vi "A170316-11_Auto -ECU.vi"() -> ()   [LabVIEW 2020]
uses:
  2e0b5f5e-2208-4490-a798-25a802626be8.vi
  Global_Variable/A170316-11.vi
  Global_Variable/Global.vi
  Database/Global1.vi
  <vilib>/addons/database/Connection.llb/DB Tools Open Connec (String).vi
  <vilib>/addons/database/NI_Database_API.lvlib
  <vilib>/regexp/Match Regular Expression.xnode
panel:
  out "请拾取O型圈":bool
  out "请拾取弹簧":bool
  in  "控制器支架":T1(ring)
  in  "ECU步骤":T2(ring)
  in  "电机步骤":T3(ring)
  out "产品型号":string
  in  "更换产品":refnum<vi>
  in  "前序OK？_ECU":string
  in  "前序OK？":string
  in  "Process":string[](array[string])
  in  "Code":string[](array[string])
  in  "User":string[](array[string])
  in  "Result":string[](array[string])
  in  "Device":string[](array[string])
  out "安装支架螺栓4拧紧确认":bool
  in  "STEP2":string
  in  "STEP1":string
  out "控制器安装螺栓3拧紧确认":bool
  out "电机安装螺栓3扭矩确认":bool
  out "控制器支架螺栓5拧紧确认":bool
  out "安装扎带并取走工件":bool
  out "涂色标":bool
  out "按启动按钮拍照确认":bool
  out "电机安装螺栓2扭矩确认":bool
  out "电机安装螺栓1扭矩确认":bool
  out "安装支架涂色标":bool
  out "控制器安装螺栓2拧紧确认":bool
  out "控制器安装螺栓1拧紧确认":bool
  out "安装支架螺栓2拧紧确认":bool
  out "安装弹性垫圈弹簧并按启动拍照":bool
  out "安装支架螺栓1拧紧确认":bool
  out "控制器支架涂色标":bool
  out "控制器支架螺栓4拧紧确认":bool
  out "控制器支架螺栓3拧紧确认":bool
  out "控制器支架螺栓2拧紧确认":bool
  out "控制器支架螺栓1拧紧确认":bool
  out "安装支架螺栓3拧紧确认":bool
  in  "更换布局":string
  out "安装扎带和线卡并取走工件":bool
  out "安装支架扎带安装":bool
  out "安装支架线卡扎带安装":bool
  out "控制器支架安装线卡扎带":bool
  out "磨合次数":i32
  in  "判定结果":bool[][](array[boolean])=[[TRUE]]
  in  "STEP3":string
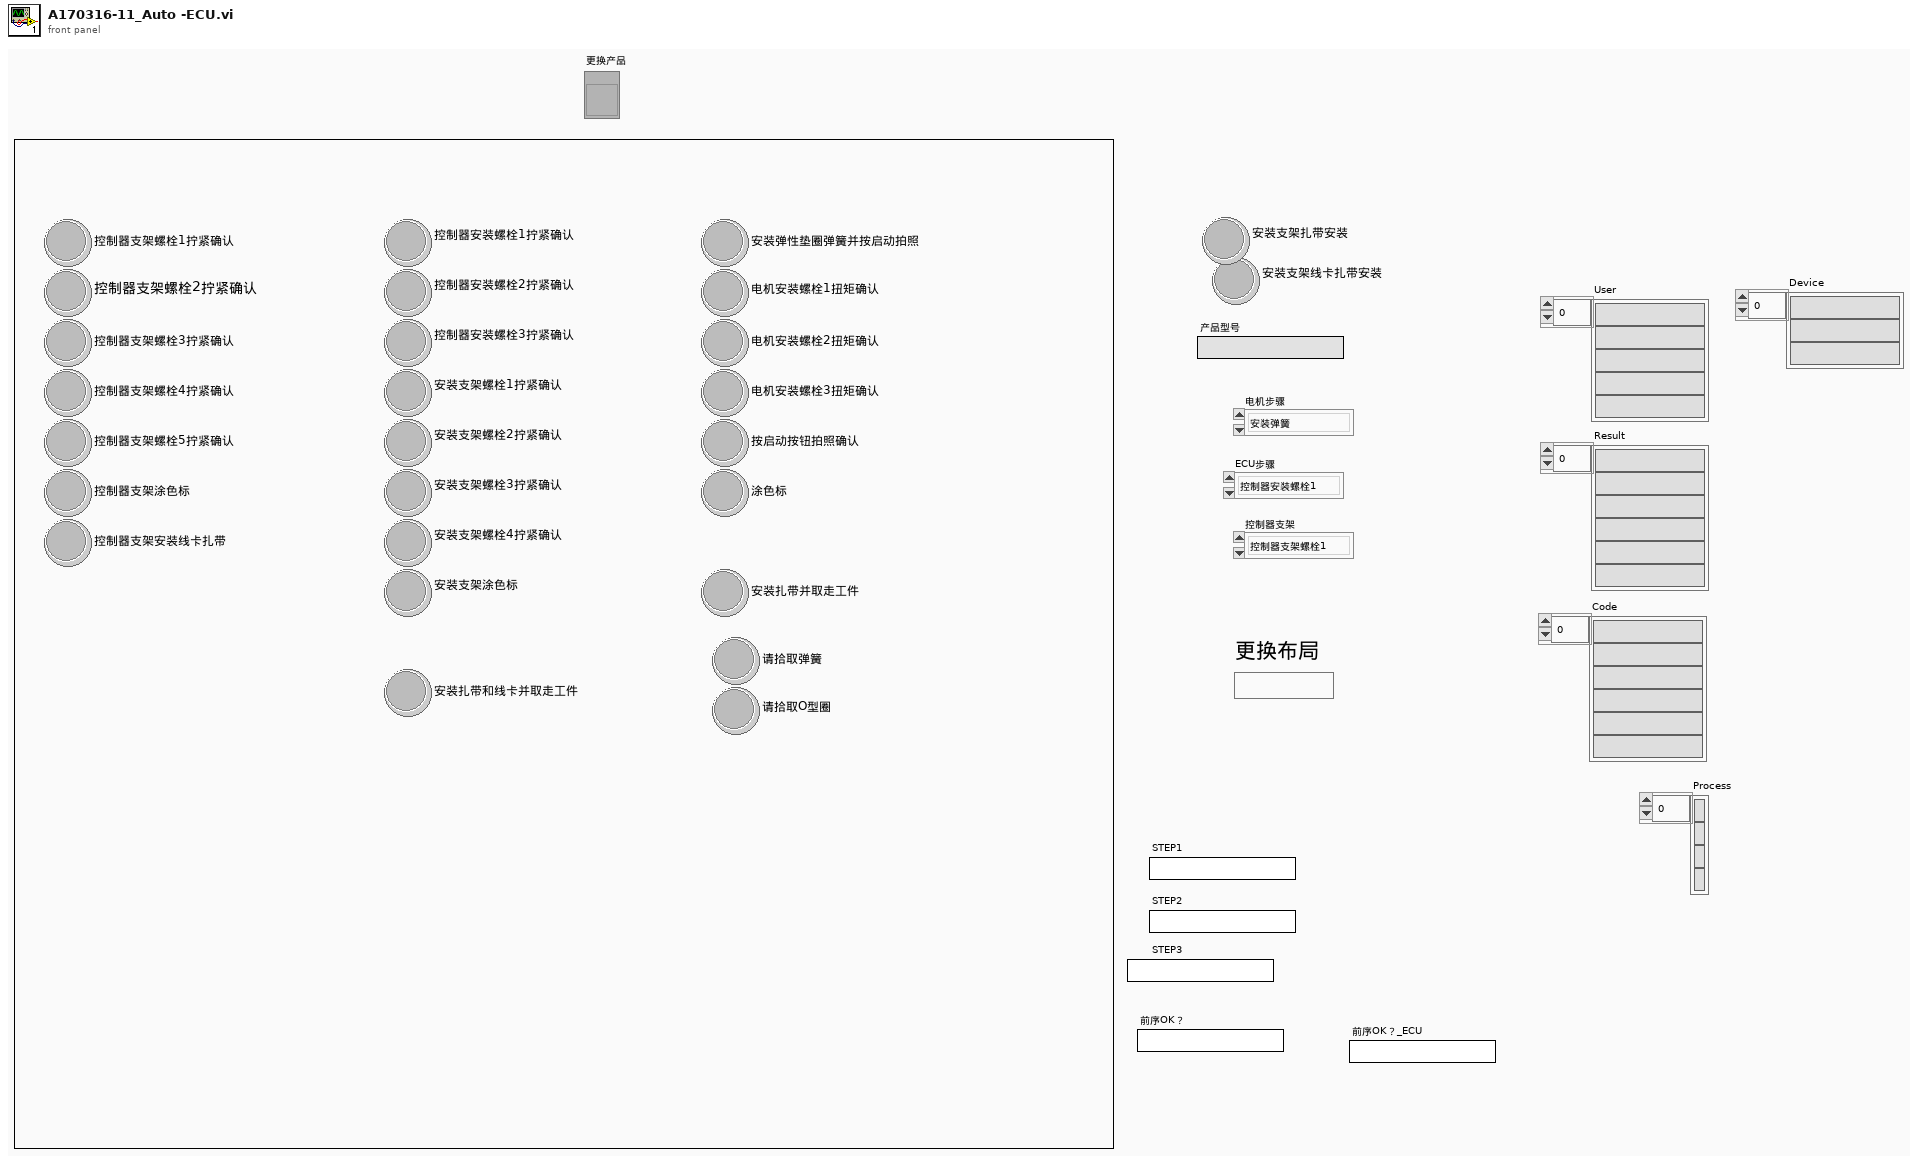
[diagram p1: front panel]
types:
  T1 = enum16{"控制器支架螺栓1", "控制器支架螺栓2", "控制器支架螺栓3", "控制器支架螺栓4", "控制器支架螺栓5", "涂色标", "安装线卡轧带", "完成"}
  T2 = enum16{"控制器安装螺栓1", "控制器安装螺栓2", "控制器安装螺栓3", "安装支架螺栓1", "安装支架螺栓2", "安装支架螺栓3", "安装支架螺栓4", "涂色标", "安装线卡取走工件", "完成"}
  T3 = enum16{"安装弹簧", "安装O型圈", "安装弹性垫圈", "电机螺栓1", "电机螺栓2", "电机螺栓3", "电机拍照", "涂色标", "安装轧带取走工件", "完成"}
  T4 = cluster{i64, i64, i64, "ECU工位生产结果":string, "result string":string}
  T5 = cluster{i64, i64, i64, "ECU工位生产结果":string, "result string":string}[]
  T6 = typedef "NI_Database_API.lvlib/Conn ObjectReference.ctl" = refnum<k1>
  T7 = cluster{"ECU工位生产结果":string, "result string":string}
  T8 = cluster{i64, i64, i64, "电机工位生产结果":string, "result string":string}
  T9 = cluster{i64, i64, i64, "电机工位生产结果":string, "result string":string}[]
  T10 = cluster{"电机工位生产结果":string, "result string":string}
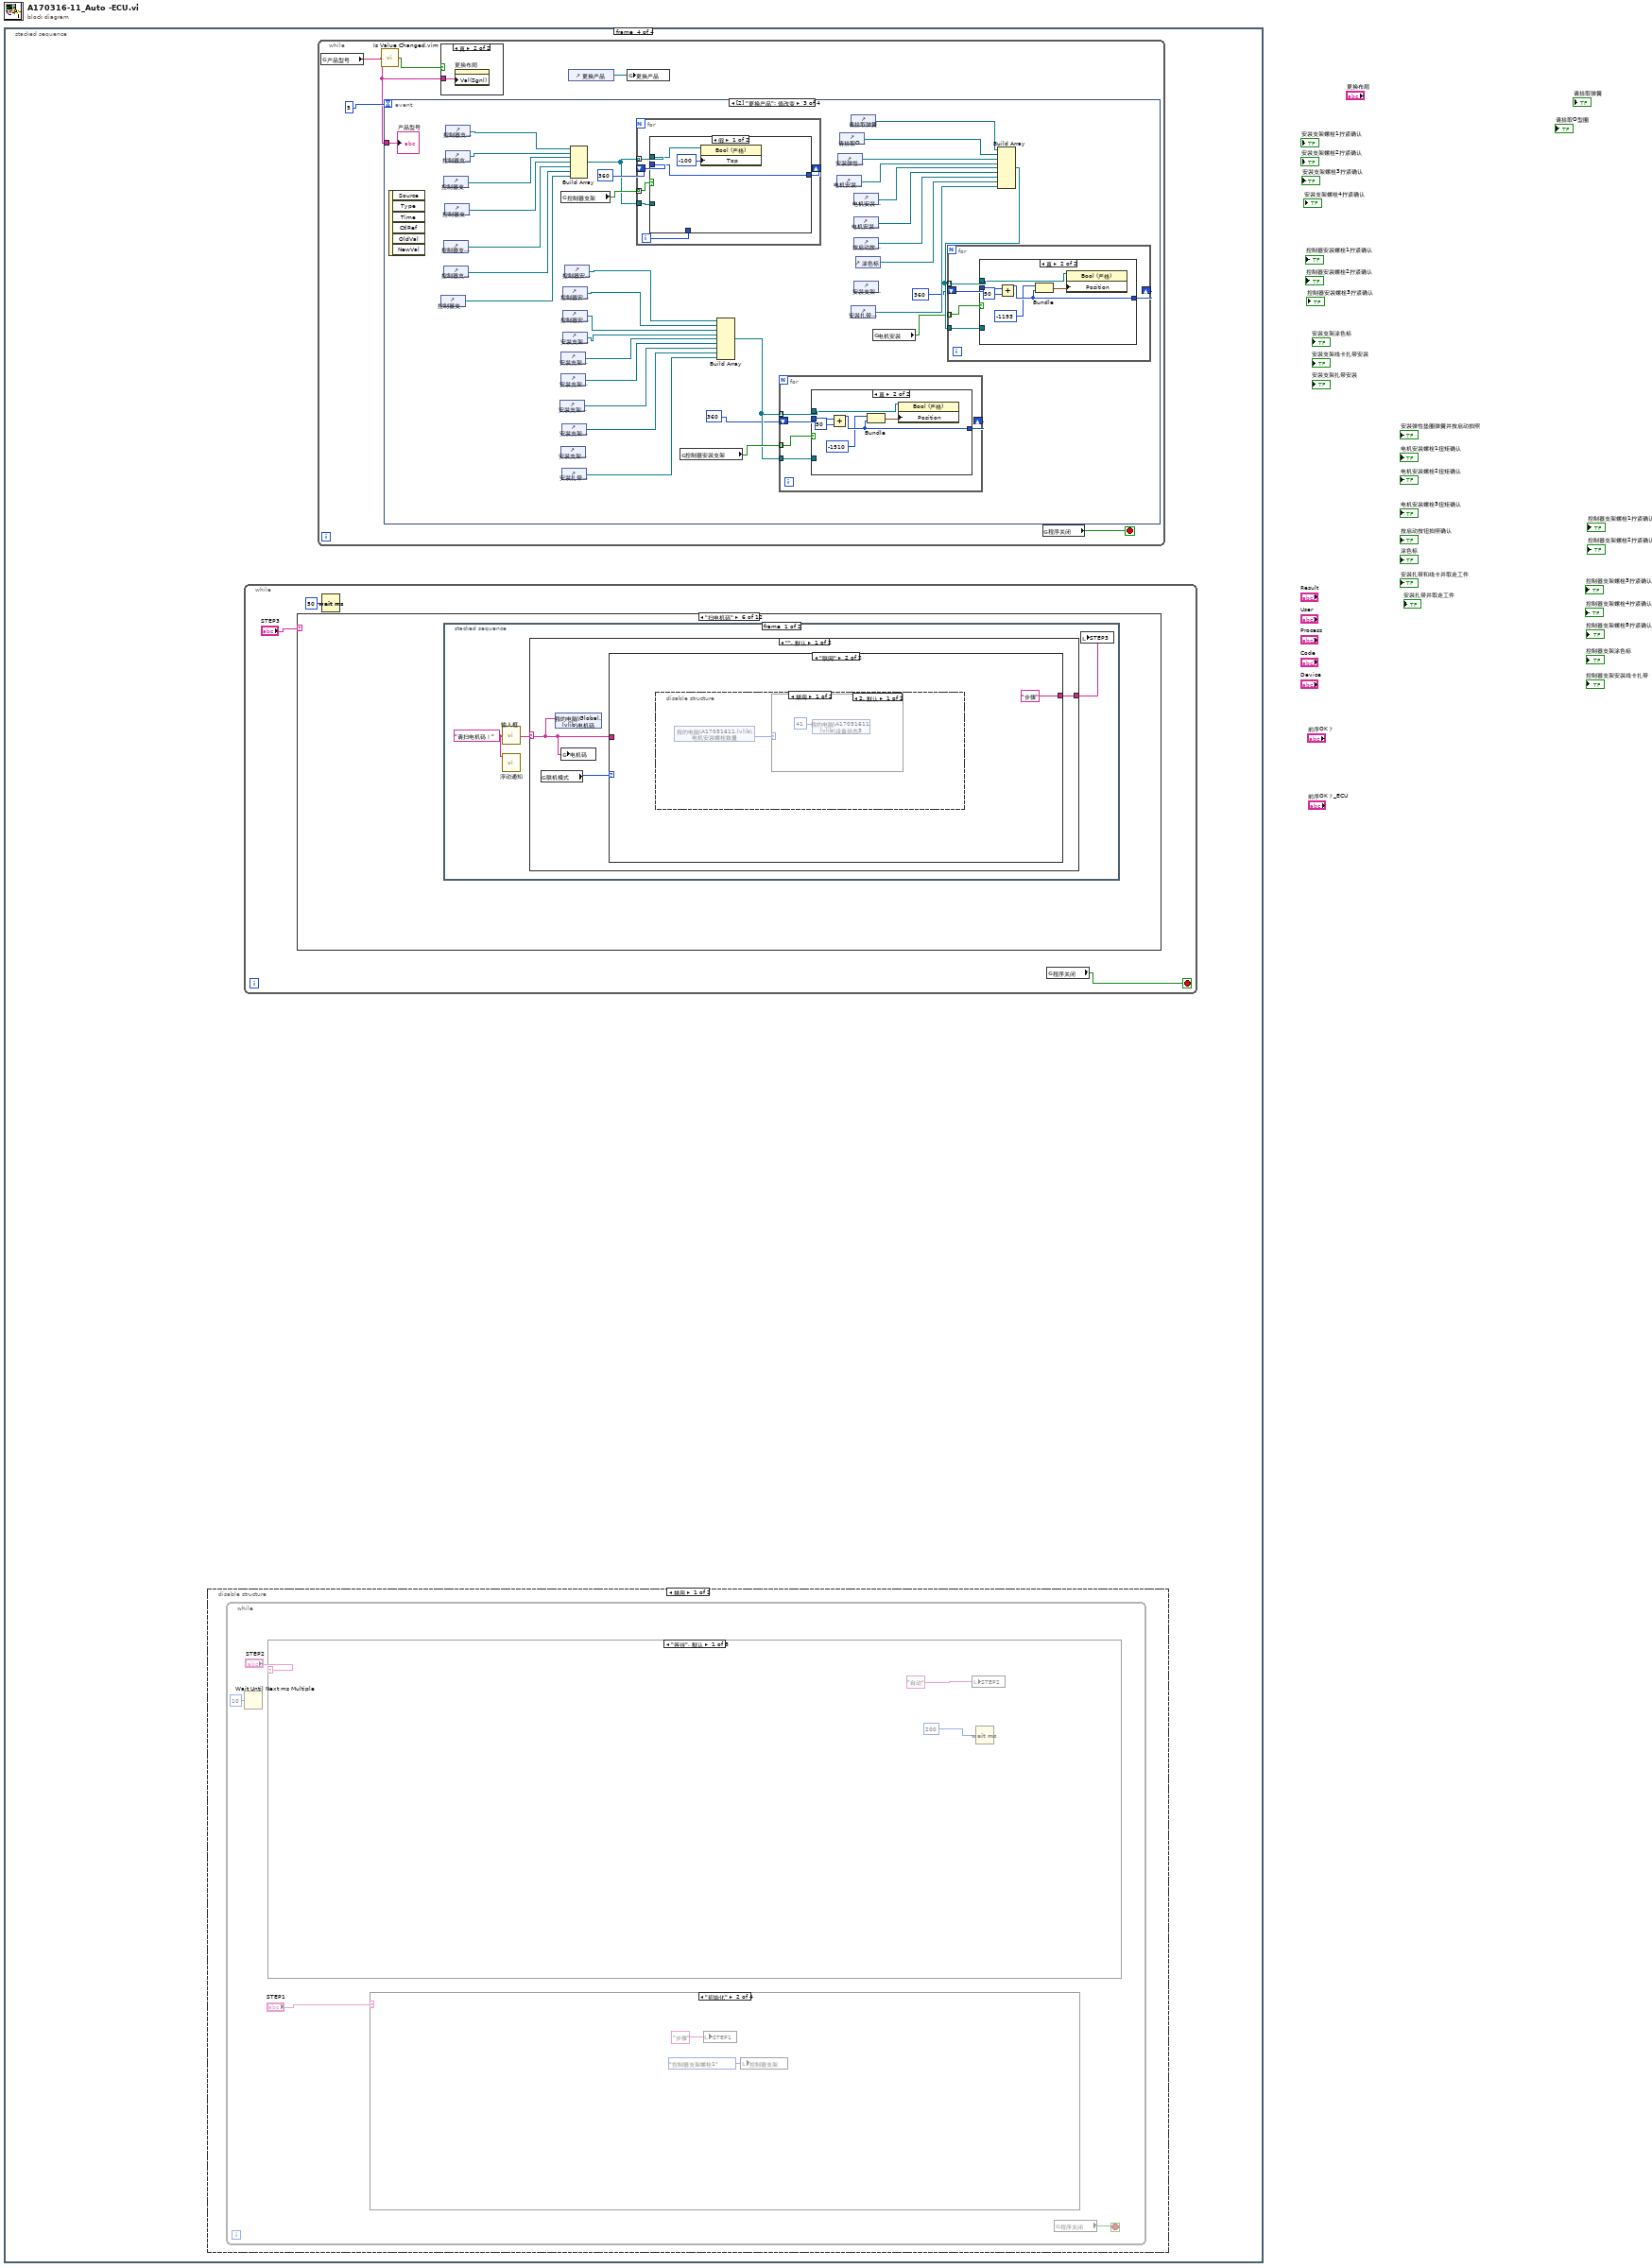
[diagram p0: block diagram]
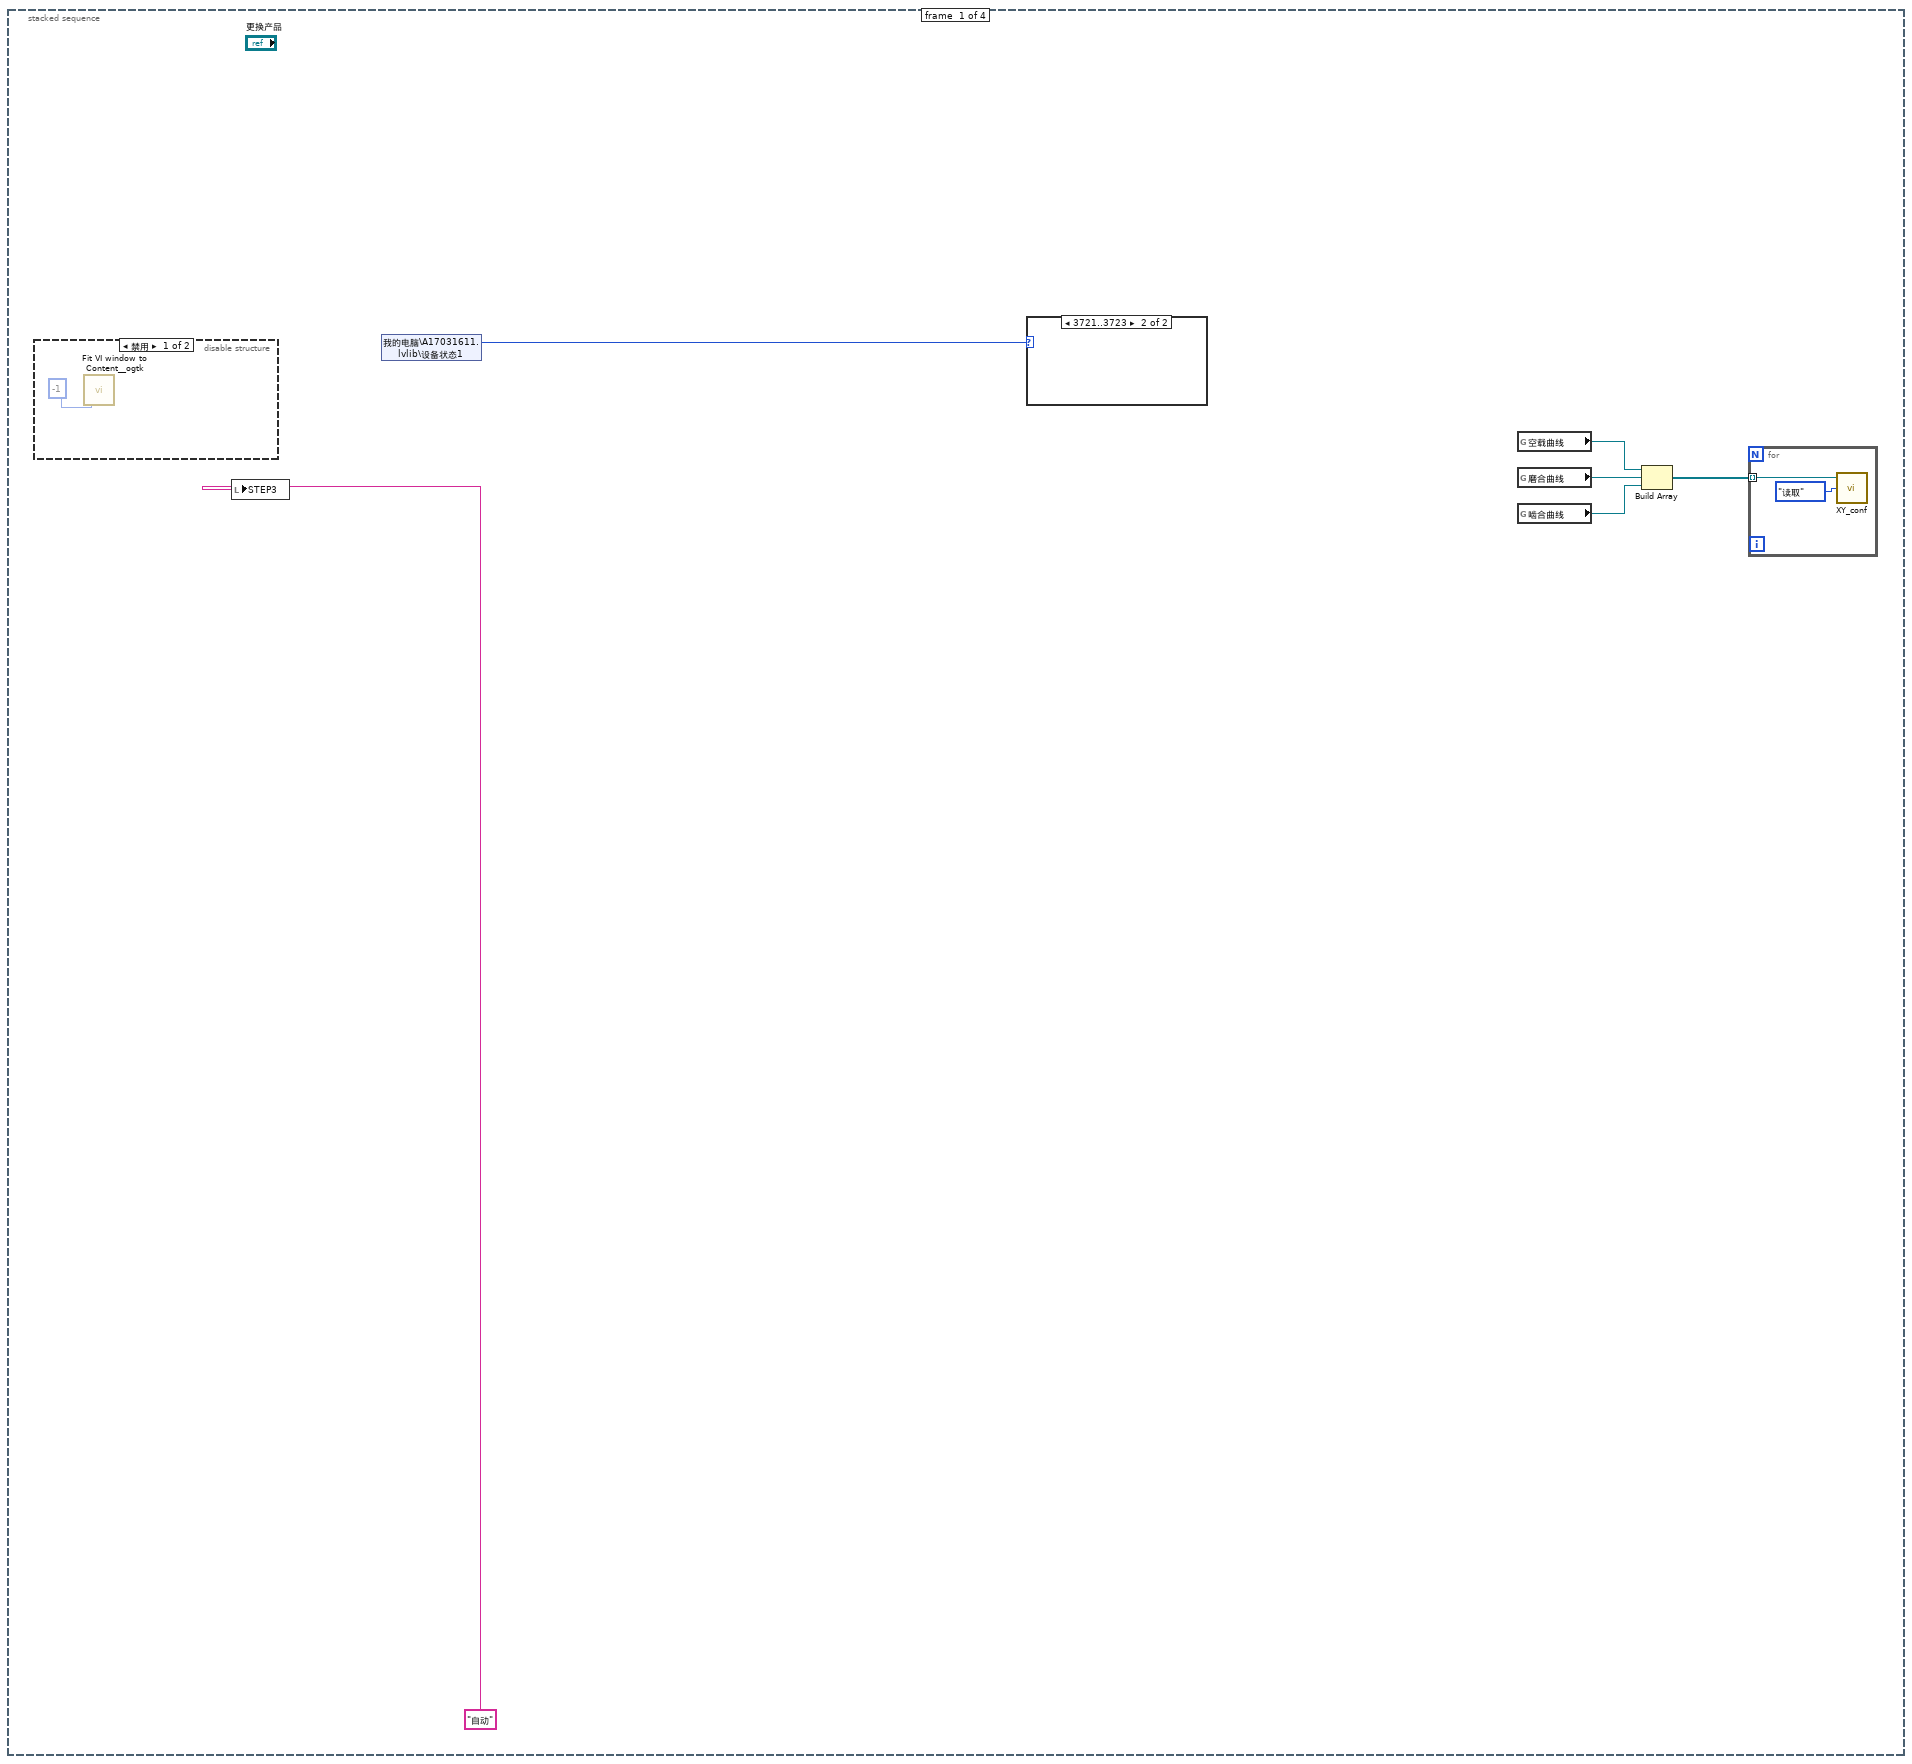
[diagram p2: hidden frame]
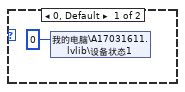
[diagram p4: hidden frame]
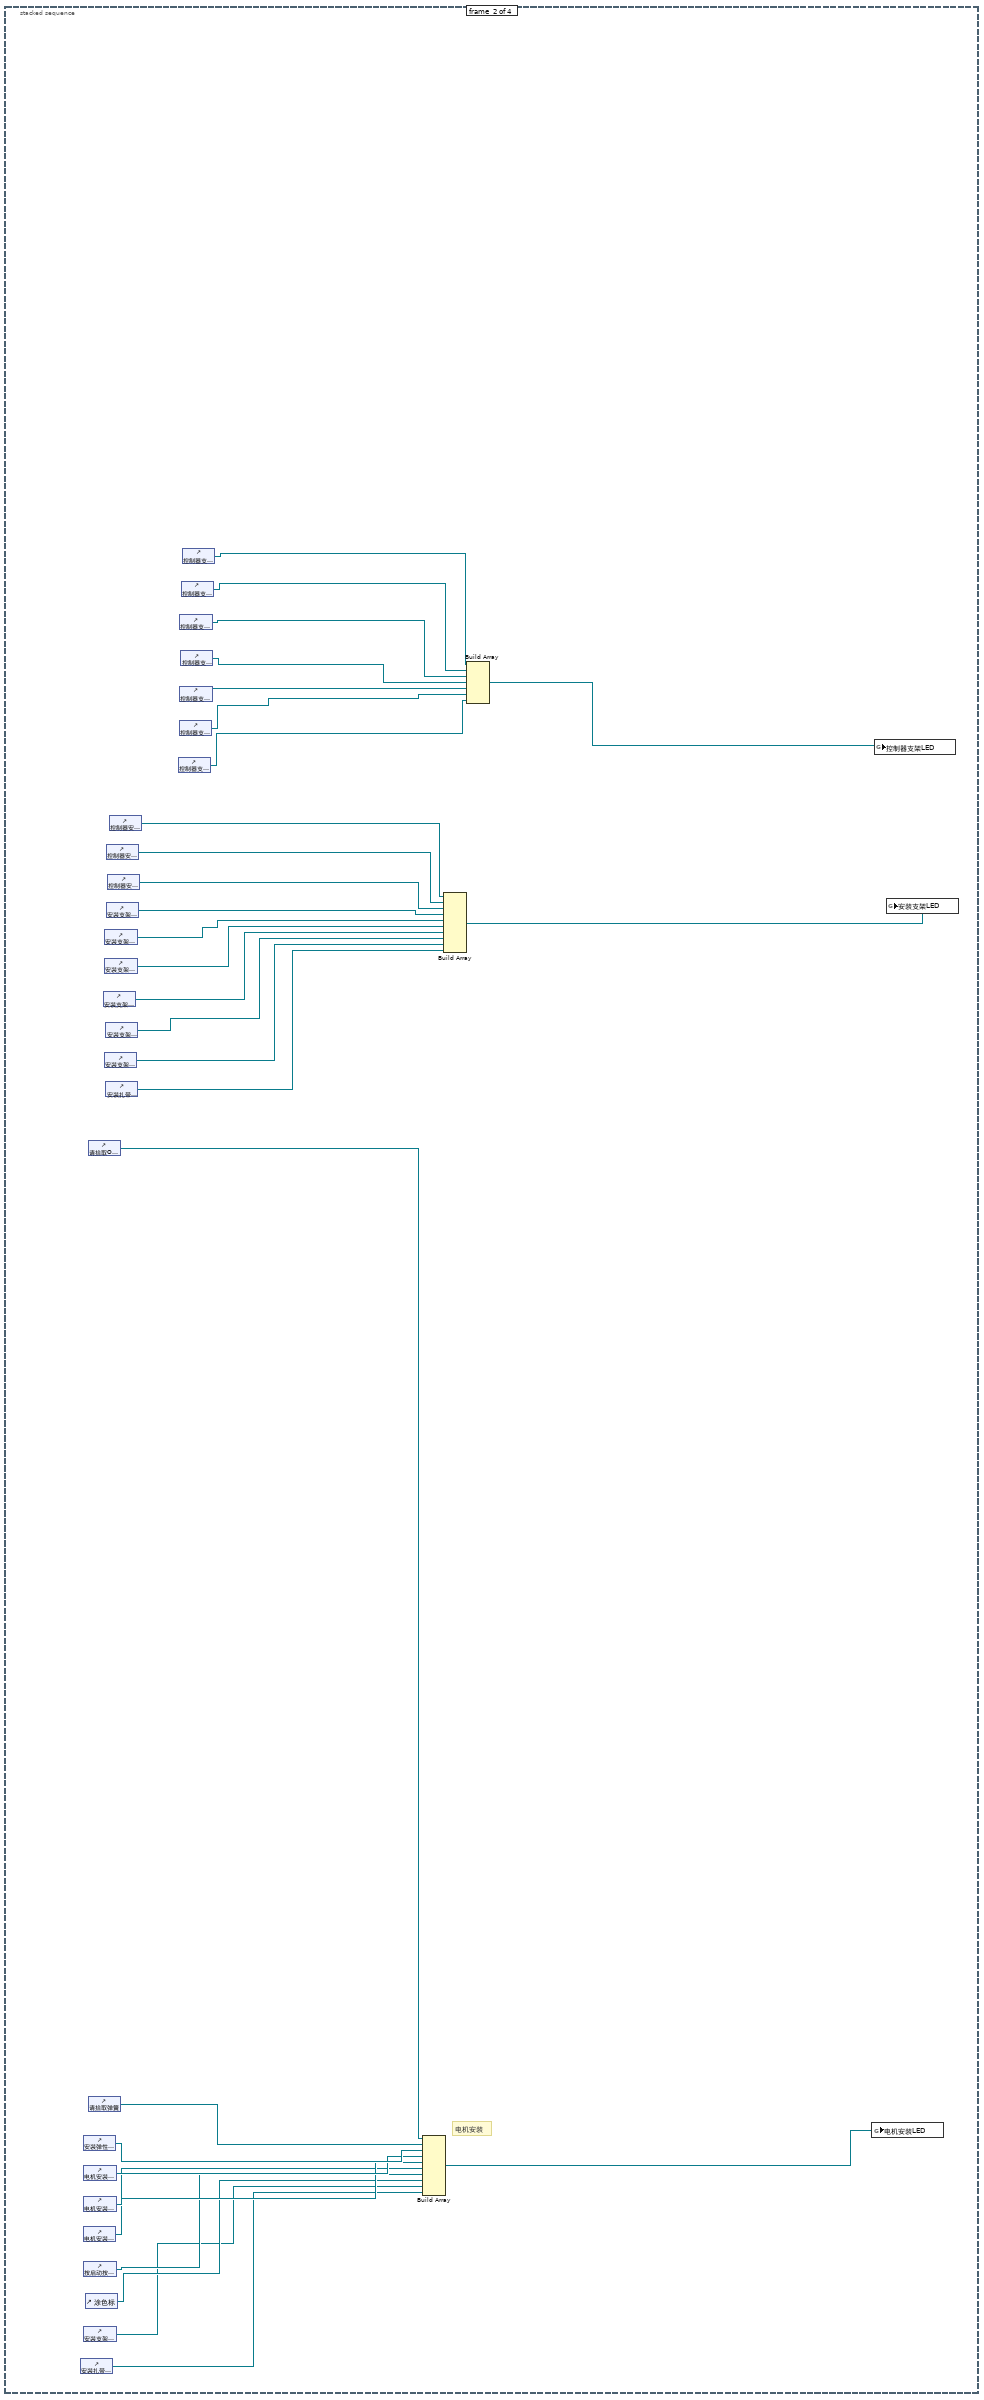
[diagram p5: hidden frame]
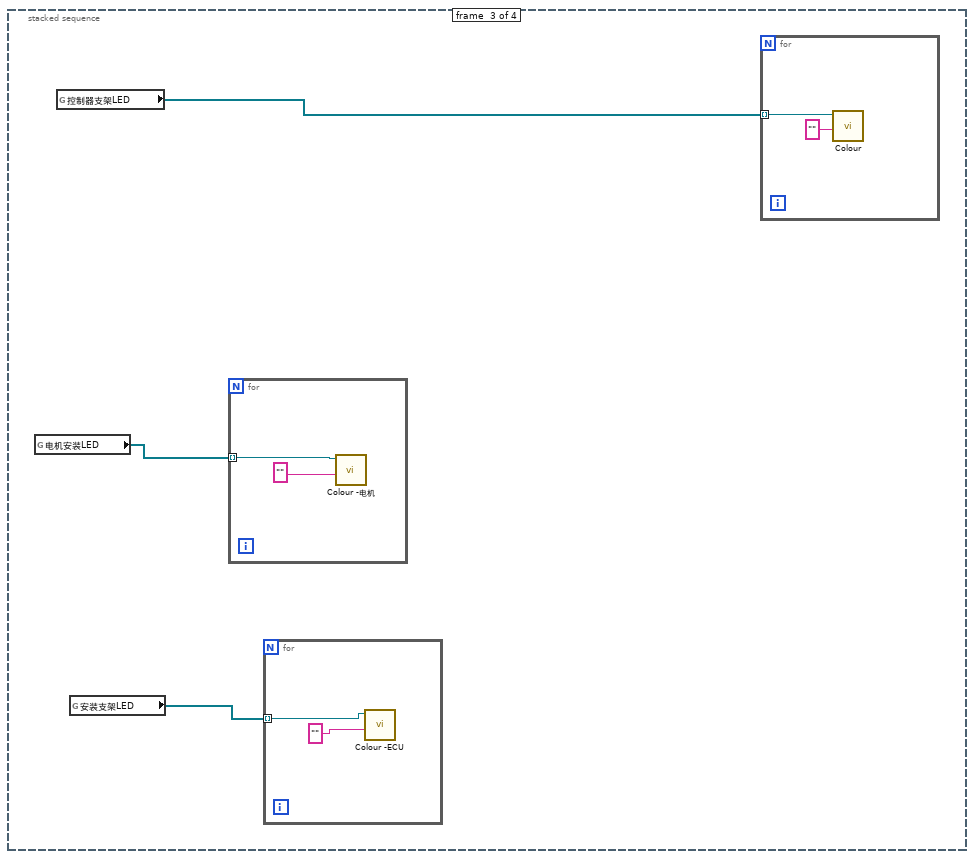
[diagram p6: hidden frame]
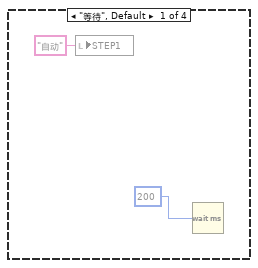
[diagram p7: hidden frame]
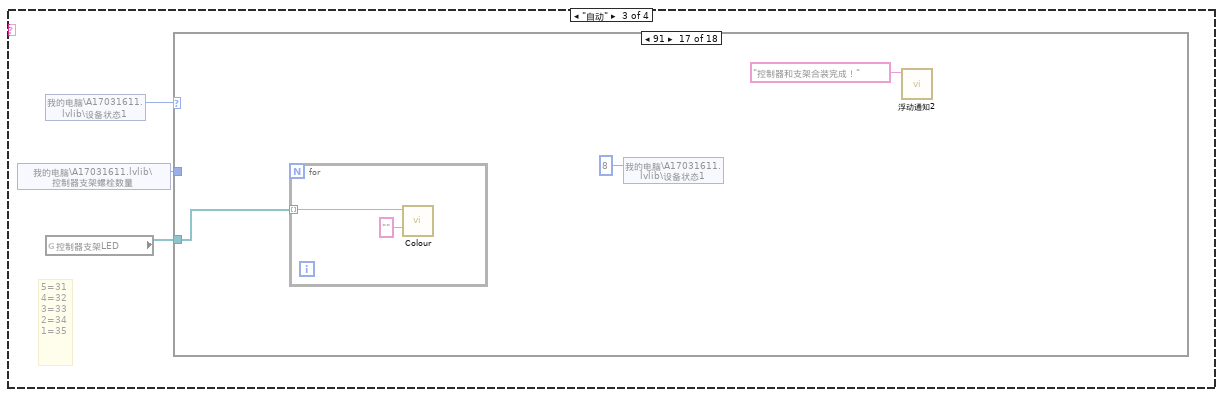
[diagram p8: hidden frame]
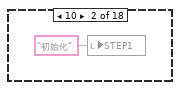
[diagram p10: hidden frame]
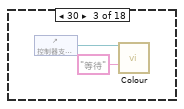
[diagram p11: hidden frame]
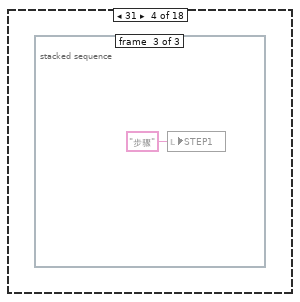
[diagram p12: hidden frame]
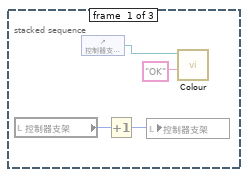
[diagram p13: hidden frame]
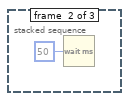
[diagram p14: hidden frame]
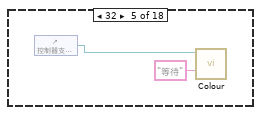
[diagram p15: hidden frame]
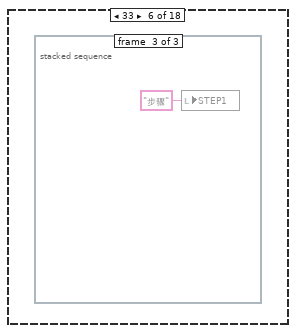
[diagram p16: hidden frame]
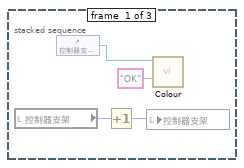
[diagram p17: hidden frame]
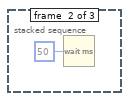
[diagram p18: hidden frame]
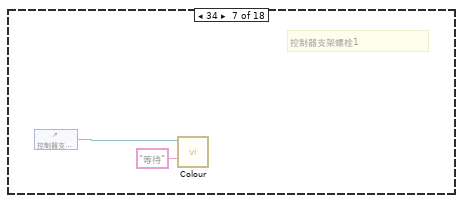
[diagram p19: hidden frame]
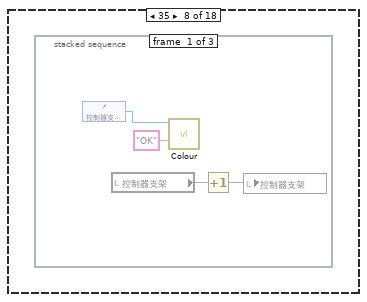
[diagram p20: hidden frame]
diagram:
  n1 = stacked-sequence {
    frame #0 {
      n2 = disable-structure shown="禁用" {
        frame Disabled {
          n3 = call "Fit VI window to Content__ogtk.vi"("border spacing (2 px)"=-1) -> ()  [unwired: 5 in, 2 out]
        }
        frame Enabled {
        }
      }
      n4 = local write "STEP3"("自动" ("STEP")) -> ()
      n5 = shared-variable "我的电脑\\A17031611.lvlib\\设备状态1"() -> (w4:i16)  [unwired: 1 in, 1 out]
      n6 = case shown="3721..3723" w4 {
        frame 0, Default {
          n7 = shared-variable "我的电脑\\A17031611.lvlib\\设备状态1"(i16 0 ("设备状态")) -> ()  [unwired: 1 in, 1 out]
        }
        frame 3721..3723 {
        }
      }
      n8 = global read "A170316-11.vi" "空载曲线"() -> (w1:refnum<vi>)
      n9 = global read "A170316-11.vi" "磨合曲线"() -> (w2:refnum<vi>)
      n10 = global read "A170316-11.vi" "啮合曲线"() -> (w3:refnum<vi>)
      n11 = Build Array(w1, w2, w3) -> (w5:refnum<vi>[])
      n12 = for {
        tunnel: w5 -> [w10] mode=indexing
        n13 = call "XY_conf.vi"("方式"=enum16{"写入", "读取"}."读取", "XY图引用"=w10) -> ()  [unwired: 3 in, 1 out]
      }
    }
    frame #1 {
      # "电机安装"
      n14 = control-ref of="安装扎带并取走工件"() -> (w23:refnum<vi>)
      n15 = control-ref of="安装弹性垫圈弹簧并按启动拍照"() -> (w30:refnum<vi>)
      n16 = control-ref of="电机安装螺栓3扭矩确认"() -> (w27:refnum<vi>)
      n17 = control-ref of="电机安装螺栓1扭矩确认"() -> (w29:refnum<vi>)
      n18 = control-ref of="电机安装螺栓2扭矩确认"() -> (w28:refnum<vi>)
      n19 = control-ref of="按启动按钮拍照确认"() -> (w26:refnum<vi>)
      n20 = control-ref of="安装支架扎带安装"() -> (w24:refnum<vi>)
      n21 = control-ref of="涂色标"() -> (w25:refnum<vi>)
      n22 = control-ref of="请拾取O型圈"() -> (w11:refnum<vi>)
      n23 = control-ref of="请拾取弹簧"() -> (w12:refnum<vi>)
      n24 = control-ref of="安装支架螺栓4拧紧确认"() -> (w16:refnum<vi>)
      n25 = control-ref of="安装支架线卡扎带安装"() -> (w14:refnum<vi>)
      n26 = control-ref of="安装支架螺栓2拧紧确认"() -> (w18:refnum<vi>)
      n27 = control-ref of="安装支架螺栓3拧紧确认"() -> (w17:refnum<vi>)
      n28 = control-ref of="安装支架涂色标"() -> (w15:refnum<vi>)
      n29 = control-ref of="安装扎带和线卡并取走工件"() -> (w13:refnum<vi>)
      n30 = control-ref of="控制器安装螺栓2拧紧确认"() -> (w21:refnum<vi>)
      n31 = control-ref of="安装支架螺栓1拧紧确认"() -> (w19:refnum<vi>)
      n32 = control-ref of="控制器安装螺栓3拧紧确认"() -> (w20:refnum<vi>)
      n33 = control-ref of="控制器安装螺栓1拧紧确认"() -> (w22:refnum<vi>)
      n34 = control-ref of="控制器支架安装线卡扎带"() -> (w31:refnum<vi>)
      n35 = control-ref of="控制器支架涂色标"() -> (w32:refnum<vi>)
      n36 = control-ref of="控制器支架螺栓3拧紧确认"() -> (w35:refnum<vi>)
      n37 = control-ref of="控制器支架螺栓5拧紧确认"() -> (w33:refnum<vi>)
      n38 = control-ref of="控制器支架螺栓4拧紧确认"() -> (w34:refnum<vi>)
      n39 = control-ref of="控制器支架螺栓2拧紧确认"() -> (w36:refnum<vi>)
      n40 = control-ref of="控制器支架螺栓1拧紧确认"() -> (w37:refnum<vi>)
      n41 = Build Array(w11, w12, w30, w29, w28, w27, w26, w25, w24, w23) -> (w40:refnum<vi>[])
      n42 = Build Array(w22, w21, w20, w19, w18, w17, w16, w15, w14, w13) -> (w39:refnum<vi>[])
      n43 = Build Array(w37, w36, w35, w34, w33, w32, w31) -> (w38:refnum<vi>[])
      n44 = global write "A170316-11.vi" "电机安装LED"(w40) -> ()
      n45 = global write "A170316-11.vi" "控制器支架LED"(w38) -> ()
      n46 = global write "A170316-11.vi" "安装支架LED"(w39) -> ()
    }
    frame #2 {
      n47 = global read "A170316-11.vi" "电机安装LED"() -> (w42:refnum<vi>[])
      n48 = global read "A170316-11.vi" "控制器支架LED"() -> (w43:refnum<vi>[])
      n49 = global read "A170316-11.vi" "安装支架LED"() -> (w41:refnum<vi>[])
      n50 = for {
        tunnel: w42 -> [w47] mode=indexing
        n51 = call "Colour -电机.vi"("result"="", "colourRef"=w47) -> ()  [unwired: 9 in, 1 out]
      }
      n52 = for {
        tunnel: w41 -> [w45] mode=indexing
        n53 = call "Colour -ECU.vi"("result"="", "colourRef"=w45) -> ()  [unwired: 9 in, 1 out]
      }
      n54 = for {
        tunnel: w43 -> [w48] mode=indexing
        n55 = call "Colour.vi"("result"="", "colourRef"=w48) -> ()  [unwired: 9 in, 1 out]
      }
    }
    frame #3 {
      n56 = disable-structure shown="禁用" {
        frame Disabled {
          n57 = while {
            stop <- w53 stop-if-true
            n58 = Wait Until Next ms Multiple(millisecond multiple=u32 10 ("毫秒倍数")) -> ()  [unwired: 1 out]
            n59 = case shown="\"等待\", 默认" "STEP2" {
              frame "等待", Default {
                n60 = local write "STEP2"("自动" ("STEP")) -> ()
                n61 = Wait (ms)(milliseconds to wait=u32 200 ("等待时间（毫秒）")) -> ()  [unwired: 1 out]
              }
              frame "手动" {
              }
              frame "初始化" {
                n62 = stacked-sequence {
                  frame #0 {
                    w179 = enum16{"录入", "清空"}."清空" ("功能")
                    n63 = global read "Global.vi" "安装支架生产数量"() -> (w171:refnum<vi>)
                    n64 = shared-variable "我的电脑\\Global.lvlib\\工位追溯码"("" ("传感器码")) -> ()  [unwired: 1 in, 1 out]
                    n65 = call "物料信息录入.vi"("功能"=w179) -> ("错误输出"=w178:errorcluster)  [unwired: 14 in]
                    n66 = call "质量信息录入.vi"("功能"=w179, "错误输入（无错误）"=w178) -> ("错误输出"=w180:errorcluster)  [unwired: 13 in]
                    n67 = property class="Num"(reference=w171, "Value"=0 ("磨合次数")) -> ()  [unwired: 1 in, 2 out]
                    n68 = call "不合格信息录入.vi"("功能"=w179, "错误输入（无错误）"=w180) -> ()  [unwired: 13 in, 1 out]
                    n69 = global read "Global.vi" "ECU自动"() -> (w176:refnum<vi>)
                    n70 = global read "Global.vi" "检测结果"() -> (w174:refnum<vi>)
                    n71 = property class="Bool (严格)"(reference=w176, "Value"=TRUE) -> ()  [unwired: 1 in, 2 out]
                    n72 = shared-variable "我的电脑\\A17031611.lvlib\\设备状态2"(i16 6 ("设备状态")) -> ()  [unwired: 1 in, 1 out]
                    n73 = call "Colour.vi"("result"="", "colourRef"=w174) -> ()  [unwired: 9 in, 1 out]
                  }
                  frame #1 {
                    n74 = local write "ECU步骤"(T2."控制器安装螺栓1" ("ECU步骤")) -> ()
                  }
                  frame #2 {
                    n75 = local write "STEP2"("等待" ("STEP2")) -> ()
                  }
                }
              }
              frame "扫主码" {
                n76 = stacked-sequence {
                  frame #0 {
                    w184 = "请扫ECU工位主码！" ("提示信息")
                    n77 = call "浮动通知2.vi"("通知内容"=w184) -> ()  [unwired: 11 in]
                    n78 = call "输入框.vi"("提示信息"=w184) -> ("条形码输出"=w185:string)
                    n79 = case shown="\"\", 默认" w185 {
                      selector: w185 -> [w186 _]
                      tunnel: [w187 "手动"] -> w183
                      frame "", Default {
                        n80 = shared-variable "我的电脑\\Global.lvlib\\工位追溯码_ECU"(w186) -> ()  [unwired: 1 in, 1 out]
                        n81 = global write "Global1.vi" "工位追溯码_ECU"(w186) -> ()
                        n82 = global read "Global1.vi" "联机模式"() -> (w188:enum16{"单机", "联网"})
                        n83 = case shown="\"联网\"" w188 {
                          tunnel: w186 -> [_ w192]
                          tunnel: ["控制器扫码" ("State(s) in Front (\"\")") w191] -> w187
                          frame "单机", Default {
                            n84 = Wait (ms)(milliseconds to wait=u32 100 ("等待时间（毫秒）")) -> ()  [unwired: 1 out]
                          }
                          frame "联网" {
                            n85 = stacked-sequence {
                              tunnel: w192 -> [w193 _ _]
                              tunnel: [_ _ w213] -> w191
                              frame #0 {
                                n86 = global read "Global1.vi" "PRODUCT_ID_ECU"() -> (w197:string)
                                n87 = Format Into String "格式化写入字符串"(format string="SELECT\ndbo.[Code].CODE_ID\nFROM\ndbo.[Code]\nWHERE\ndbo.[Code].CODE_MAIN = '%s'\nAND\ndbo.[Code].PRODUCT_ID = %s\n" ("格式字符串"), w193, w197) -> (resulting string=w199:string)  [unwired: 2 in, 1 out]
                                n88 = call "SQL_query.vi"("SQL query"=w199, "联机模式"=enum16{"单机", "联网"}."联网") -> ("data"=w202:string[][])  [unwired: 1 in, 2 out]
                                n89 = Index Array(array=w202, index (row)=0 ("索引 (行)")) -> (element=w201:string[])  [unwired: 1 in]
                                n90 = Index Array(array=w201, index=0 ("索引")) -> (element=w194:string)
                                n91 = global write "Global1.vi" "CODE_ID_ECU"(w194) -> ()
                              }
                              frame #1 {
                                n92 = global read "Global1.vi" "前序DEVICE_ID_ECU"() -> (w203:string)
                                n93 = global read "Global1.vi" "CODE_ID_ECU"() -> (w204:string)
                                n94 = Format Into String(format string="SELECT\ndbo.[Result].RESULT_VALUE\nFROM\ndbo.[Result]\nWHERE\ndbo.[Result].DEVICE_ID = %s\nAND\ndbo.[Result].CODE_ID = %s\n" ("格式字符串"), w203, w204) -> (resulting string=w206:string)  [unwired: 2 in, 1 out]
                                n95 = call "SQL_query.vi"("SQL query"=w206, "联机模式"=enum16{"单机", "联网"}."联网") -> ("data"=w212:string[][])  [unwired: 1 in, 2 out]
                                n96 = Index Array(array=w212, index (row)=0 ("索引 (行)")) -> (element=w211:string[])  [unwired: 1 in]
                                n97 = Index Array(array=w211, index=0 ("索引")) -> (element=w205:string)
                                n98 = local write "前序OK？_ECU"(w205) -> ()
                              }
                              frame #2 {
                                n99 = local read "前序OK？_ECU"() -> (w214:string)
                                n100 = case shown="\"OK\"" w214 {
                                tunnel: ["控制器扫码" "自动" "自动"] -> w213
                                frame "OK" {
                                n101 = global read "Global.vi" "ECU前序显示字"() -> (w218:refnum<vi>)
                                n102 = global read "Global1.vi" "ECU上序状态"() -> (w217:refnum<vi>)
                                n103 = property class="Str"(reference=w218, "Value"="OK" ("值")) -> ()  [unwired: 1 in, 2 out]
                                n104 = call "Colour -ECU.vi"("result"="OK", "colourRef"=w217) -> ()  [unwired: 9 in, 1 out]
                                n105 = Wait (ms)(milliseconds to wait=u32 100 ("等待时间（毫秒）")) -> ()  [unwired: 1 out]
                                }
                                frame Default {
                                n106 = global read "Global1.vi" "ECU上序状态"() -> (w224:refnum<vi>)
                                n107 = Wait (ms)(milliseconds to wait=u32 2000 ("等待时间（毫秒）")) -> ()  [unwired: 1 out]
                                n108 = call "浮动通知2.vi"("通知内容"="ECU工位上序漏序！" ("Status")) -> ()  [unwired: 11 in]
                                n109 = global read "Global.vi" "ECU前序显示字"() -> (w221:refnum<vi>)
                                n110 = call "Colour.vi"("result"="等待", "colourRef"=w224) -> ()  [unwired: 9 in, 1 out]
                                n111 = shared-variable "我的电脑\\A17031611.lvlib\\设备状态2"(i16 6 ("设备状态控制字")) -> ()  [unwired: 1 in, 1 out]
                                n112 = property class="Str"(reference=w221, "Value"="漏序" ("值")) -> ()  [unwired: 1 in, 2 out]
                                }
                                frame "NG" {
                                n113 = Wait (ms)(milliseconds to wait=u32 2000 ("等待时间（毫秒）")) -> ()  [unwired: 1 out]
                                n114 = global read "Global1.vi" "ECU上序状态"() -> (w230:refnum<vi>)
                                n115 = call "浮动通知2.vi"("通知内容"="上序生产结果不合格！" ("Status")) -> ()  [unwired: 11 in]
                                n116 = global read "Global.vi" "ECU前序显示字"() -> (w232:refnum<vi>)
                                n117 = call "Colour -ECU.vi"("result"="NG", "colourRef"=w230) -> ()  [unwired: 9 in, 1 out]
                                n118 = shared-variable "我的电脑\\A17031611.lvlib\\设备状态2"(i16 6 ("设备状态控制字")) -> ()  [unwired: 1 in, 1 out]
                                n119 = property class="Str"(reference=w232, "Value"="NG" ("值")) -> ()  [unwired: 1 in, 2 out]
                                }
                                }
                              }
                            }
                          }
                        }
                      }
                      frame "exit" {
                      }
                    }
                    n120 = local write "STEP2"(w183) -> ()
                  }
                  frame #1 {
                    n121 = Wait (ms)(milliseconds to wait=u32 100 ("等待时间（毫秒）")) -> ()  [unwired: 1 out]
                  }
                }
              }
              frame "控制器扫码" {
                n122 = stacked-sequence {
                  frame #0 {
                    w239 = "请扫请控制器码！！" ("提示信息")
                    n123 = call "输入框.vi"("提示信息"=w239) -> ("条形码输出"=w240:string)
                    n124 = call "浮动通知2.vi"("通知内容"=w239) -> ()  [unwired: 11 in]
                    n125 = case shown="\"\", 默认" w240 {
                      selector: w240 -> [w246 _]
                      tunnel: [w249 "手动"] -> w241
                      frame "", Default {
                        n126 = global read "Global.vi" "硬件版本号"() -> (w242:string)
                        n127 = global write "Global1.vi" "控制器码"(w246) -> ()
                        n128 = shared-variable "我的电脑\\Global.lvlib\\控制器码"(w246) -> ()  [unwired: 1 in, 1 out]
                        n129 = xnode "匹配正则表达式"("输入字符串"=w246, "正则表达式"="-") -> ("匹配之前"=w244:string)  [unwired: 4 in, 4 out]
                        n130 = call <vilib>:"Trim Whitespace.vi"("string"=w244) -> ("trimmed string"=w247:string)  [unwired: 1 in]
                        n131 = call <vilib>:"Trim Whitespace.vi"("string"=w242) -> ("trimmed string"=w248:string)  [unwired: 1 in]
                        n132 = Equal?(x=w247, y=w248) -> (x = y?=w243:bool)
                        n133 = case shown="真" w243 {
                          tunnel: ["控制器扫码" ("State(s) in Front (\"\")") w369] -> w249
                          frame False {
                            w367 = 0 items=["OK", "OKCancel", "AbortRetryIgnore", "YesNoCancel", "YesNo", "RetryCancel"] ("buttons")
                            w368 = 16 items=["None"=0, "Hand, Error, Stop"=16, "Question"=32, "Exclamation, Warning"=48, "Asterisk, Information"=64] ("icon")
                            n134 = call "信息框（标题、文本、图标）.vi"("icon"=w368, "buttons"=w367, "caption"="控制器混料", "text"="混料请核对控制器!") -> ()  [unwired: 6 in, 2 out]
                          }
                          frame True {
                            n135 = global read "Global1.vi" "联机模式"() -> (w370:enum16{"单机", "联网"})
                            n136 = case shown="\"联网\"" w370 {
                              tunnel: ["步骤" ("State(s) in Front (\"\")") "步骤"] -> w369
                              frame "单机", Default {
                                n137 = global read "Global.vi" "安装支架生产数量"() -> (w374:refnum<vi>)
                                n138 = property class="Num"(reference=w374) -> (reference out=w375:refnum<vi>, error out=w376:errorcluster, "Value"=w377:variant)  [unwired: 1 in]
                                n139 = Variant To Data(type=u32 0, Variant=w377) -> (data=w378:u32)  [unwired: 1 in, 1 out]
                                n140 = Increment(x=w378) -> (x+1=w379:u32)
                                n141 = property class="Num"(reference=w375, error in=w376, "Value"=w379) -> ()  [unwired: 2 out]
                                n142 = Wait (ms)(milliseconds to wait=u32 10 ("等待时间（毫秒）")) -> ()  [unwired: 1 out]
                              }
                              frame "联网" {
                                n143 = global read "Global.vi" "安装支架生产数量"() -> (w382:refnum<vi>)
                                n144 = property class="Num"(reference=w382) -> (reference out=w383:refnum<vi>, error out=w384:errorcluster, "Value"=w385:variant)  [unwired: 1 in]
                                n145 = Variant To Data "变体至数据转换"(type=u32 0, Variant=w385) -> (data=w386:u32)  [unwired: 1 in, 1 out]
                                n146 = Wait (ms)(milliseconds to wait=u32 100 ("等待时间（毫秒）")) -> ()  [unwired: 1 out]
                                n147 = Increment(x=w386) -> (x+1=w387:u32)
                                n148 = property class="Num"(reference=w383, error in=w384, "Value"=w387) -> ()  [unwired: 2 out]
                              }
                            }
                          }
                        }
                      }
                      frame "exit" {
                      }
                    }
                    n149 = local write "STEP2"(w241) -> ()
                  }
                  frame #1 {
                    n150 = Wait (ms)(milliseconds to wait=u32 100 ("等待时间（毫秒）")) -> ()  [unwired: 1 out]
                  }
                }
              }
              frame "自动" {
                # "3=41\n2=42\n1=43\n0=45"
                # "4=31\n3=32\n2=33\n1=34\n0=35"
                n151 = shared-variable "我的电脑\\A17031611.lvlib\\安装支架螺栓2"() -> (w391:u16)  [unwired: 1 in, 1 out]
                n152 = shared-variable "我的电脑\\A17031611.lvlib\\安装支架螺栓数"() -> (w392:u16)  [unwired: 1 in, 1 out]
                n153 = shared-variable "我的电脑\\A17031611.lvlib\\设备状态2"() -> (w393:i16)  [unwired: 1 in, 1 out]
                n154 = global read "A170316-11.vi" "安装支架LED"() -> (w394:refnum<vi>[])
                n155 = case shown="45" w393 {
                  tunnel: w394 -> [_ _ _ _ _ w398 _ w406 _ _ _ _ _ _ _ _ _ _ _ _ _ _ _ w479 w481 _ _ w499 w502 w509 _ _ w534 _ _ _ _]
                  tunnel: w392 -> [_ _ _ _ _ _ _ w407 _ _ _ _ _ _ _ _ _ _ _ _ _ _ _ _ _ _ _ _ _ _ _ _ _ _ _ _ _]
                  tunnel: w391 -> [_ _ _ _ _ _ _ _ _ _ _ _ _ _ _ _ _ _ _ _ _ _ _ _ _ _ _ _ _ _ _ _ _ _ _ _ _]
                  frame Default {
                  }
                  frame -128 {
                    n156 = global read "Global.vi" "ECU自动"() -> (w396:refnum<vi>)
                    n157 = property class="Bool (严格)"(reference=w396, "Value"=FALSE) -> ()  [unwired: 1 in, 2 out]
                  }
                  frame 5 {
                    (unwired) "ECU工位复位完成！" ("Status")
                  }
                  frame 6 {
                    n158 = call "浮动通知2.vi"("通知内容"="请按启动确认扫ECU工位主码") -> ()  [unwired: 11 in]
                  }
                  frame 0 {
                    (unwired) "手动状态！" ("Status")
                  }
                  frame 7 {
                    n159 = for {
                      tunnel: w398 -> [w405] mode=indexing
                      n160 = call "Colour -ECU.vi"("result"="", "colourRef"=w405) -> ()  [unwired: 9 in, 1 out]
                    }
                    n161 = global read "Global.vi" "ECU结果显示"() -> (w400:refnum<vi>)
                    n162 = property class="Str"(reference=w400, "Value"="..." ("结果显示")) -> (reference out=w401:refnum<vi>)  [unwired: 1 in, 1 out]
                    n163 = property class="Str"(reference=w401, "Text.TextColor"=u32 16776960) -> ()  [unwired: 1 in, 2 out]
                    n164 = local write "STEP2"("扫主码" ("STEP2")) -> ()
                  }
                  frame 9 {
                  }
                  frame 10 {
                    n165 = case shown="2" w407 {
                      tunnel: w406 -> [_ _ _ _ _]
                      frame 0, Default {
                        n166 = shared-variable "我的电脑\\A17031611.lvlib\\设备状态2"(i16 35 ("设备状态")) -> ()  [unwired: 1 in, 1 out]
                      }
                      frame 1 {
                        n167 = shared-variable "我的电脑\\A17031611.lvlib\\设备状态2"(i16 34 ("设备状态")) -> ()  [unwired: 1 in, 1 out]
                      }
                      frame 2 {
                        n168 = shared-variable "我的电脑\\A17031611.lvlib\\设备状态2"(i16 33 ("设备状态")) -> ()  [unwired: 1 in, 1 out]
                      }
                      frame 3 {
                        n169 = shared-variable "我的电脑\\A17031611.lvlib\\设备状态2"(i16 32 ("设备状态")) -> ()  [unwired: 1 in, 1 out]
                      }
                      frame 4 {
                        n170 = shared-variable "我的电脑\\A17031611.lvlib\\设备状态2"(i16 31 ("设备状态")) -> ()  [unwired: 1 in, 1 out]
                      }
                    }
                  }
                  frame 31 {
                    n171 = control-ref of="控制器安装螺栓1拧紧确认"() -> (w414:refnum<vi>)
                    n172 = call "浮动通知2.vi"("通知内容"="请安装固定螺栓1并确认扭矩！" ("Status")) -> ()  [unwired: 11 in]
                    n173 = call "Colour -ECU.vi"("result"="等待", "colourRef"=w414) -> ()  [unwired: 9 in, 1 out]
                  }
                  frame 32 {
                    n174 = stacked-sequence {
                      frame #0 {
                        n175 = local read "ECU步骤"() -> (w417:T2)
                        n176 = control-ref of="控制器安装螺栓1拧紧确认"() -> (w418:refnum<vi>)
                        n177 = Increment(x=w417) -> (x+1=w416:T2)
                        n178 = local write "ECU步骤"(w416) -> ()
                        n179 = call "Colour.vi"("result"="OK", "colourRef"=w418) -> ()  [unwired: 9 in, 1 out]
                      }
                      frame #1 {
                        n180 = Wait (ms)(milliseconds to wait=u32 50 ("等待时间（毫秒）")) -> ()  [unwired: 1 out]
                      }
                      frame #2 {
                        n181 = local write "STEP2"("步骤" ("STEP2")) -> ()
                      }
                    }
                  }
                  frame 33 {
                    n182 = control-ref of="控制器安装螺栓2拧紧确认"() -> (w423:refnum<vi>)
                    n183 = call "浮动通知2.vi"("通知内容"="控制器安装螺栓2拧紧确认！" ("Status")) -> ()  [unwired: 11 in]
                    n184 = call "Colour -ECU.vi"("result"="等待", "colourRef"=w423) -> ()  [unwired: 9 in, 1 out]
                  }
                  frame 34 {
                    n185 = stacked-sequence {
                      frame #0 {
                        n186 = local read "ECU步骤"() -> (w426:T2)
                        n187 = control-ref of="控制器安装螺栓2拧紧确认"() -> (w428:refnum<vi>)
                        n188 = Increment(x=w426) -> (x+1=w425:T2)
                        n189 = local write "ECU步骤"(w425) -> ()
                        n190 = call "Colour -ECU.vi"("result"="OK", "colourRef"=w428) -> ()  [unwired: 9 in, 1 out]
                      }
                      frame #1 {
                        n191 = Wait (ms)(milliseconds to wait=u32 50 ("等待时间（毫秒）")) -> ()  [unwired: 1 out]
                      }
                      frame #2 {
                        n192 = local write "STEP2"("步骤" ("STEP2")) -> ()
                      }
                    }
                  }
                  frame 35 {
                    n193 = control-ref of="控制器安装螺栓3拧紧确认"() -> (w432:refnum<vi>)
                    n194 = call "浮动通知2.vi"("通知内容"="控制器安装螺栓3拧紧确认!") -> ()  [unwired: 11 in]
                    n195 = call "Colour -ECU.vi"("result"="等待", "colourRef"=w432) -> ()  [unwired: 9 in, 1 out]
                  }
                  frame 36 {
                    n196 = stacked-sequence {
                      frame #0 {
                        n197 = control-ref of="控制器安装螺栓3拧紧确认"() -> (w437:refnum<vi>)
                        n198 = local read "ECU步骤"() -> (w434:T2)
                        n199 = Increment(x=w434) -> (x+1=w435:T2)
                        n200 = call "Colour -ECU.vi"("result"="等待", "colourRef"=w437) -> ()  [unwired: 9 in, 1 out]
                        n201 = local write "ECU步骤"(w435) -> ()
                      }
                      frame #1 {
                        n202 = Wait (ms)(milliseconds to wait=u32 50 ("等待时间（毫秒）")) -> ()  [unwired: 1 out]
                      }
                      frame #2 {
                        n203 = local write "STEP2"("步骤" ("STEP2")) -> ()
                      }
                    }
                  }
                  frame 40 {
                  }
                  frame 41 {
                    n204 = control-ref of="安装支架螺栓1拧紧确认"() -> (w441:refnum<vi>)
                    n205 = call "Colour -ECU.vi"("result"="等待", "colourRef"=w441) -> ()  [unwired: 9 in, 1 out]
                    n206 = call "浮动通知2.vi"("通知内容"="请安装控制器支架1并确认扭矩！" ("Status")) -> ()  [unwired: 11 in]
                  }
                  frame 42 {
                    n207 = stacked-sequence {
                      frame #0 {
                        n208 = local read "ECU步骤"() -> (w443:T2)
                        n209 = control-ref of="安装支架螺栓1拧紧确认"() -> (w446:refnum<vi>)
                        n210 = Increment(x=w443) -> (x+1=w444:T2)
                        n211 = local write "ECU步骤"(w444) -> ()
                        n212 = call "Colour -ECU.vi"("result"="OK", "colourRef"=w446) -> ()  [unwired: 9 in, 1 out]
                      }
                      frame #1 {
                        n213 = Wait (ms)(milliseconds to wait=u32 50 ("等待时间（毫秒）")) -> ()  [unwired: 1 out]
                      }
                      frame #2 {
                        n214 = local write "STEP2"("步骤" ("STEP2")) -> ()
                      }
                    }
                  }
                  frame 43 {
                    n215 = control-ref of="安装支架螺栓2拧紧确认"() -> (w450:refnum<vi>)
                    n216 = call "Colour -ECU.vi"("result"="等待", "colourRef"=w450) -> ()  [unwired: 9 in, 1 out]
                    n217 = call "浮动通知2.vi"("通知内容"="请安装控制器支架2并确认扭矩！" ("Status")) -> ()  [unwired: 11 in]
                  }
                  frame 44 {
                    n218 = stacked-sequence {
                      frame #0 {
                        n219 = local read "ECU步骤"() -> (w453:T2)
                        n220 = control-ref of="安装支架螺栓2拧紧确认"() -> (w455:refnum<vi>)
                        n221 = Increment(x=w453) -> (x+1=w452:T2)
                        n222 = call "Colour -ECU.vi"("result"="OK", "colourRef"=w455) -> ()  [unwired: 9 in, 1 out]
                        n223 = local write "ECU步骤"(w452) -> ()
                      }
                      frame #1 {
                        n224 = Wait (ms)(milliseconds to wait=u32 50 ("等待时间（毫秒）")) -> ()  [unwired: 1 out]
                      }
                      frame #2 {
                        n225 = local write "STEP2"("步骤" ("STEP2")) -> ()
                      }
                    }
                  }
                  frame 45 {
                    n226 = control-ref of="安装支架螺栓3拧紧确认"() -> (w459:refnum<vi>)
                    n227 = call "浮动通知2.vi"("通知内容"="请安装控制器支架3并确认扭矩") -> ()  [unwired: 11 in]
                    n228 = call "Colour -ECU.vi"("result"="等待", "colourRef"=w459) -> ()  [unwired: 9 in, 1 out]
                  }
                  frame 46 {
                    n229 = stacked-sequence {
                      frame #0 {
                        n230 = local read "ECU步骤"() -> (w462:T2)
                        n231 = control-ref of="安装支架螺栓3拧紧确认"() -> (w464:refnum<vi>)
                        n232 = Increment(x=w462) -> (x+1=w461:T2)
                        n233 = local write "ECU步骤"(w461) -> ()
                        n234 = call "Colour -ECU.vi"("result"="OK", "colourRef"=w464) -> ()  [unwired: 9 in, 1 out]
                      }
                      frame #1 {
                        n235 = Wait (ms)(milliseconds to wait=u32 50 ("等待时间（毫秒）")) -> ()  [unwired: 1 out]
                      }
                      frame #2 {
                        n236 = local write "STEP2"("步骤" ("STEP2")) -> ()
                      }
                    }
                  }
                  frame 47 {
                    n237 = control-ref of="安装支架螺栓4拧紧确认"() -> (w468:refnum<vi>)
                    n238 = call "浮动通知2.vi"("通知内容"="请安装控制器支架4并确认扭矩") -> ()  [unwired: 11 in]
                    n239 = call "Colour -ECU.vi"("result"="等待", "colourRef"=w468) -> ()  [unwired: 9 in, 1 out]
                  }
                  frame 48 {
                    n240 = stacked-sequence {
                      frame #0 {
                        n241 = control-ref of="安装支架螺栓4拧紧确认"() -> (w473:refnum<vi>)
                        n242 = local read "ECU步骤"() -> (w471:T2)
                        n243 = Increment(x=w471) -> (x+1=w470:T2)
                        n244 = local write "ECU步骤"(w470) -> ()
                        n245 = call "Colour -ECU.vi"("result"="OK", "colourRef"=w473) -> ()  [unwired: 9 in, 1 out]
                      }
                      frame #1 {
                        n246 = Wait (ms)(milliseconds to wait=u32 50 ("等待时间（毫秒）")) -> ()  [unwired: 1 out]
                      }
                      frame #2 {
                        n247 = local write "STEP2"("步骤" ("STEP2")) -> ()
                      }
                    }
                  }
                  frame 60 {
                    n248 = Index Array(array=w479, index=4 ("索引")) -> ()  [unwired: 1 out]
                    n249 = call "浮动通知2.vi"("通知内容"="请取记号笔标记!") -> ()  [unwired: 11 in]
                    n250 = control-ref of="安装支架涂色标"() -> (w477:refnum<vi>)
                    n251 = call "Colour -ECU.vi"("result"="等待", "colourRef"=w477) -> ()  [unwired: 9 in, 1 out]
                  }
                  frame 61 {
                    n252 = Index Array(array=w481, index #1=4 ("索引")) -> ()  [unwired: 1 in, 2 out]
                    n253 = stacked-sequence {
                      frame #0 {
                        n254 = control-ref of="安装支架涂色标"() -> (w485:refnum<vi>)
                        n255 = local read "ECU步骤"() -> (w484:T2)
                        n256 = Increment(x=w484) -> (x+1=w483:T2)
                        n257 = local write "ECU步骤"(w483) -> ()
                        n258 = call "Colour.vi"("result"="OK", "colourRef"=w485) -> ()  [unwired: 9 in, 1 out]
                      }
                      frame #1 {
                        n259 = Wait (ms)(milliseconds to wait=u32 50 ("等待时间（毫秒）")) -> ()  [unwired: 1 out]
                      }
                      frame #2 {
                        n260 = local write "STEP2"("步骤" ("STEP2")) -> ()
                      }
                    }
                  }
                  frame 70 {
                    n261 = control-ref of="安装支架线卡扎带安装"() -> (w490:refnum<vi>)
                    n262 = call "Colour -ECU.vi"("result"="等待", "colourRef"=w490) -> ()  [unwired: 9 in, 1 out]
                    n263 = call "浮动通知2.vi"("通知内容"="请取轧带！" ("Status")) -> ()  [unwired: 11 in]
                  }
                  frame 81 {
                    n264 = stacked-sequence {
                      frame #0 {
                        n265 = local read "ECU步骤"() -> (w493:T2)
                        n266 = control-ref of="安装支架线卡扎带安装"() -> (w496:refnum<vi>)
                        n267 = Increment(x=w493) -> (x+1=w492:T2)
                        n268 = local write "ECU步骤"(w492) -> ()
                        n269 = call "浮动通知2.vi"("通知内容"="完成！" ("Status")) -> ()  [unwired: 11 in]
                        n270 = call "Colour -ECU.vi"("result"="OK", "colourRef"=w496) -> ()  [unwired: 9 in, 1 out]
                      }
                      frame #1 {
                        n271 = Wait (ms)(milliseconds to wait=u32 50 ("等待时间（毫秒）")) -> ()  [unwired: 1 out]
                      }
                      frame #2 {
                        n272 = local write "STEP2"("步骤" ("STEP2")) -> ()
                      }
                    }
                  }
                  frame 71 {
                    n273 = Index Array(array=w499, index #1=8 ("索引")) -> ()  [unwired: 1 in, 2 out]
                    n274 = shared-variable "我的电脑\\A17031611.lvlib\\设备状态2"(i16 200 ("设备状态")) -> ()  [unwired: 1 in, 1 out]
                  }
                  frame 91 {
                    (unwired) "请安装电机扎带并取走工件！" ("Status")
                    n275 = Index Array(array=w502, index #1=5 ("索引")) -> (element #1=w504:refnum<vi>, element #2=w503:refnum<vi>)  [unwired: 1 in]
                    n276 = call "Colour.vi"("result"="OK", "colourRef"=w504) -> ()  [unwired: 9 in, 1 out]
                    n277 = call "Colour.vi"("result"="等待", "colourRef"=w503) -> ()  [unwired: 9 in, 1 out]
                    n278 = shared-variable "我的电脑\\A17031611.lvlib\\设备状态3"(i16 100 ("设备状态")) -> ()  [unwired: 1 in, 1 out]
                  }
                  frame 101 {
                    (unwired) "完成！" ("Status")
                    n279 = Index Array(array=w509, index #1=6 ("索引")) -> (element #1=w511:refnum<vi>, element #2=w510:refnum<vi>)  [unwired: 1 in]
                    n280 = call "Colour.vi"("result"="OK", "colourRef"=w511) -> ()  [unwired: 9 in, 1 out]
                    n281 = call "Colour.vi"("result"="等待", "colourRef"=w510) -> ()  [unwired: 9 in, 1 out]
                    n282 = shared-variable "我的电脑\\A17031611.lvlib\\设备状态3"(i16 110 ("设备状态")) -> ()  [unwired: 1 in, 1 out]
                  }
                  frame 200 {
                    n283 = global read "Global.vi" "检测结果"() -> (w525:refnum<vi>)
                    n284 = global write "Global1.vi" "ECU工位生产结果"("OK" ("电机工位生产结果")) -> ()
                    n285 = call "浮动通知2.vi"("通知内容"="产品合格！" ("Status")) -> ()  [unwired: 11 in]
                    n286 = call "Colour.vi"("result"="OK", "colourRef"=w525) -> ()  [unwired: 9 in, 1 out]
                    n287 = global read "Global.vi" "ECU结果显示"() -> (w523:refnum<vi>)
                    n288 = property class="Str"(reference=w523, "Value"="OK" ("结果显示")) -> (reference out=w520:refnum<vi>)  [unwired: 1 in, 1 out]
                    n289 = global read "Global1.vi" "联机模式"() -> (w517:enum16{"单机", "联网"})
                    n290 = property class="Str"(reference=w520, "Text.TextColor"=u32 6618880) -> ()  [unwired: 1 in, 2 out]
                    n291 = case shown="\"单机\", 默认" w517 {
                      tunnel: ["初始化" "录入数据库" ("STEP3")] -> w516
                      frame "单机", Default {
                      }
                      frame "联网" {
                      }
                    }
                    n292 = local write "STEP2"(w516) -> ()
                  }
                  frame 201 {
                    (unwired) "产品不合格！" ("Status")
                    n293 = global read "Global.vi" "检测结果"() -> (w532:refnum<vi>)
                    n294 = call "Colour.vi"("result"="NG", "colourRef"=w532) -> ()  [unwired: 9 in, 1 out]
                    n295 = global read "Global.vi" "电机结果显示"() -> (w531:refnum<vi>)
                    n296 = property class="Str"(reference=w531, "Value"="NG" ("结果显示")) -> (reference out=w530:refnum<vi>)  [unwired: 1 in, 1 out]
                    n297 = property class="Str"(reference=w530, "Text.TextColor"=u32 16711680) -> ()  [unwired: 1 in, 2 out]
                  }
                  frame 999 {
                    n298 = for {
                      tunnel: w534 -> [w537] mode=indexing
                      n299 = call "Colour.vi"("result"="", "colourRef"=w537) -> ()  [unwired: 9 in, 1 out]
                    }
                    n300 = call "浮动通知2.vi"("通知内容"="请重新安装固定螺栓！" ("Status")) -> ()  [unwired: 11 in]
                    n301 = shared-variable "我的电脑\\A17031611.lvlib\\设备状态2"(i16 31 ("设备状态")) -> ()  [unwired: 1 in, 1 out]
                  }
                  frame 1024 {
                    n302 = global read "Global.vi" "ECU自动"() -> (w540:refnum<vi>)
                    n303 = property class="Bool (严格)"(reference=w540, "Value"=FALSE) -> ()  [unwired: 1 in, 2 out]
                  }
                  frame 3721 {
                    (unwired) "产品不合格程序锁定！" ("Status")
                    n304 = local write "STEP3"("不合格锁定" ("STEP")) -> ()
                  }
                  frame 3722 {
                    n305 = global read "Global.vi" "ECU自动"() -> (w543:refnum<vi>)
                    n306 = property class="Bool (严格)"(reference=w543, "Value"=FALSE) -> ()  [unwired: 1 in, 2 out]
                  }
                  frame 3723 {
                    (unwired) "请取出不合格产品并摆放至不合格品区！" ("Status")
                  }
                }
              }
              frame "录入数据库" {
                n307 = stacked-sequence {
                  frame #0 {
                    n308 = Get Date/Time String(date format (0)=enum16{"short", "long", "abbreviated"}."short" ("日期格式(0)"), want seconds? (F)=FALSE ("需要秒？(F)")) -> (date string=w553:string, time string=w554:string)  [unwired: 1 in]
                    n309 = global read "Global1.vi" "DEVICE_ID_ECU"() -> (w557:string)
                    n310 = global read "Global1.vi" "CODE_ID_ECU"() -> (w556:string)
                    n311 = global read "Global1.vi" "ECU工位生产结果"() -> (w548:string)
                    n312 = global read "Global1.vi" "USER_ID"() -> (w555:string)
                    n313 = Concatenate Strings(w553, " " ("字符串"), w554) -> (w549:string)
                    n314 = Decimal String To Number(string=w557, default (0L)=i64 0 ("默认(0 I32)")) -> (number=w546:i64)  [unwired: 1 in, 1 out]
                    n315 = Decimal String To Number(string=w555, default (0L)=i64 0 ("默认(0 I32)")) -> (number=w545:i64)  [unwired: 1 in, 1 out]
                    n316 = Decimal String To Number(string=w556, default (0L)=i64 0 ("默认(0 I32)")) -> (number=w544:i64)  [unwired: 1 in, 1 out]
                    n317 = global read "Global1.vi" "联机模式"() -> (w564:enum16{"单机", "联网"})
                    n318 = Search and Replace String(replace all?=TRUE ("替换全部？(F)"), input string=w549, search string="/" ("替换字符串(\"\")"), replace string="-" ("替换字符串(\"\")")) -> (result string=w547:string)  [unwired: 4 in, 3 out]
                    n319 = Bundle(w546, w545, w544, "ECU工位生产结果"=w548, "result string"=w547) -> (w570:T4)  [unwired: 1 in]
                    n320 = call "GetSQLstring.vi"("联机模式"=w564) -> ("错误输出"=w567:errorcluster, "连接字符串"=w566:string)  [unwired: 9 in]
                    n321 = Build Array(w570) -> (w571:T5)
                    n322 = call-poly <vilib>:"DB Tools Open Connection.vi"("error in (no error)"=w567, "connection information"=w566) -> ("error out"=w565:errorcluster, "connection reference"=w568:T6)  [unwired: 6 in]
                    n323 = for {
                      tunnel: w571 -> [w576] mode=indexing
                      tunnel: w568 -> [w574]
                      shift-right: [w572] -> w569
                      shift-left: w565 -> [w579]
                      w575 = string[] ["DEVICE_ID", "USER_ID", "CODE_ID", "RESULT_VALUE", "RESULT_TIME"] ("columns")
                      w577 = "Result" ("table")
                      n324 = call <vilib>:"DB Tools Insert Data.vi"("data"=w576, "error in (no error)"=w579, "columns"=w575, "table"=w577, "connection reference"=w574) -> ("error out"=w578:errorcluster, "connection reference out"=w573:T6)  [unwired: 5 in]
                      n325 = case shown="错误" w578 {
                        selector: w578 -> [w580 w601]
                        tunnel: w575 -> [_ w598]
                        tunnel: w573 -> [w581 w590]
                        tunnel: w577 -> [_ w602]
                        tunnel: w576 -> [_ w594]
                        tunnel: [w581 w589] -> _
                        tunnel: [w580 w588] -> w572
                        frame No Error {
                        }
                        frame Error {
                          n326 = Array Subset(array=w598, index=3 ("长度"), length=2 ("长度")) -> (w599:string[])
                          n327 = Unbundle(w594) -> (w583:i64, w586:i64, "ECU工位生产结果"=w593:string, "result string"=w592:string)  [unwired: 1 out]
                          n328 = Number To Decimal String(number=w586) -> (decimal integer string=w587:string)  [unwired: 1 in]
                          n329 = Number To Decimal String(number=w583) -> (decimal integer string=w582:string)  [unwired: 1 in]
                          n330 = Concatenate Strings("WHERE CODE_ID =" ("condition"), w587, "AND DEVICE_ID = ", w582) -> (w595:string)
                          n331 = Bundle("ECU工位生产结果"=w593, "result string"=w592) -> (w591:T7)  [unwired: 1 in]
                          n332 = call <vilib>:"Clear Errors.vi"("error in (no error)"=w601) -> ("error out"=w600:errorcluster)  [unwired: 5 in, 1 out]
                          n333 = call <vilib>:"DB Tools Update Data.vi"("condition"=w595, "data"=w591, "error in (no error)"=w600, "columns"=w599, "table"=w602, "connection reference"=w590) -> ("error out"=w588:errorcluster, "connection reference out"=w589:T6)  [unwired: 4 in]
                        }
                      }
                    }
                    n334 = call <vilib>:"Simple Error Handler.vi"("error in (no error)"=w569) -> ()  [unwired: 4 in, 5 out]
                  }
                  frame #1 {
                    n335 = global read "Global1.vi" "CODE_ID_ECU"() -> (w604:string)
                    n336 = global read "Global1.vi" "控制器码"() -> (w603:string)
                    n337 = Format Into String(format string="UPDATE\ndbo.[Code]\nSET dbo.[Code].CODE_ECU = '%s'\n\nWHERE\ndbo.[Code].CODE_ID = %s\n" ("格式字符串"), w603, w604) -> (resulting string=w607:string)  [unwired: 2 in, 1 out]
                    n338 = call "SQL_query.vi"("SQL query"=w607, "联机模式"=enum16{"单机", "联网"}."联网") -> ()  [unwired: 1 in, 3 out]
                  }
                  frame #2 {
                    n339 = call "浮动通知2.vi"("通知内容"="ECU工位数据录入成功！" ("Status")) -> ()  [unwired: 11 in]
                    n340 = local write "STEP2"("初始化" ("STEP2")) -> ()
                  }
                }
              }
              frame "步骤" {
                n341 = case shown="\"控制器安装螺栓1\", 默认" "ECU步骤" {
                  selector: "ECU步骤" -> [w613 _]
                  tunnel: [w612 "等待"] -> w610
                  frame "控制器安装螺栓1", Default {
                    n342 = global read "Global.vi" "控制器安装支架"() -> (w615:bool[])
                    n343 = Index Array(array=w615, index=w613) -> (element=w614:bool)
                    n344 = case shown="真" w614 {
                      tunnel: w613 -> [_ w621]
                      tunnel: ["步骤" w620] -> w612
                      frame False {
                        n345 = local read "ECU步骤"() -> (w619:T2)
                        n346 = Increment(x=w619) -> (x+1=w618:T2)
                        n347 = Wait (ms)(milliseconds to wait=u32 100 ("等待时间（毫秒）")) -> ()  [unwired: 1 out]
                        n348 = local write "ECU步骤"(w618) -> ()
                      }
                      frame True {
                        n349 = case shown="\"控制器安装螺栓1\", 默认" w621 {
                          tunnel: ["等待" "等待" "等待" "等待" "等待" "等待" "等待" "等待" "等待"] -> w620
                          frame "控制器安装螺栓1", Default {
                            n350 = shared-variable "我的电脑\\A17031611.lvlib\\设备状态2"(i16 31 ("设备状态控制字")) -> ()  [unwired: 1 in, 1 out]
                          }
                          frame "控制器安装螺栓2" {
                            n351 = shared-variable "我的电脑\\A17031611.lvlib\\设备状态2"(i16 33 ("设备状态控制字")) -> ()  [unwired: 1 in, 1 out]
                          }
                          frame "控制器安装螺栓3" {
                            n352 = shared-variable "我的电脑\\A17031611.lvlib\\设备状态2"(i16 35 ("设备状态控制字")) -> ()  [unwired: 1 in, 1 out]
                          }
                          frame "安装支架螺栓1" {
                            n353 = shared-variable "我的电脑\\A17031611.lvlib\\设备状态2"(i16 41 ("设备状态控制字")) -> ()  [unwired: 1 in, 1 out]
                          }
                          frame "安装支架螺栓2" {
                            n354 = shared-variable "我的电脑\\A17031611.lvlib\\设备状态2"(i16 43 ("设备状态控制字")) -> ()  [unwired: 1 in, 1 out]
                          }
                          frame "安装支架螺栓3" {
                            n355 = shared-variable "我的电脑\\A17031611.lvlib\\设备状态2"(i16 45 ("设备状态控制字")) -> ()  [unwired: 1 in, 1 out]
                          }
                          frame "安装支架螺栓4" {
                            n356 = shared-variable "我的电脑\\A17031611.lvlib\\设备状态2"(i16 47 ("设备状态控制字")) -> ()  [unwired: 1 in, 1 out]
                          }
                          frame "涂色标" {
                            n357 = shared-variable "我的电脑\\A17031611.lvlib\\设备状态2"(i16 60 ("设备状态控制字")) -> ()  [unwired: 1 in, 1 out]
                          }
                          frame "安装线卡取走工件" {
                            n358 = shared-variable "我的电脑\\A17031611.lvlib\\设备状态2"(i16 70 ("设备状态控制字")) -> ()  [unwired: 1 in, 1 out]
                          }
                        }
                      }
                    }
                  }
                  frame "完成" {
                    n359 = shared-variable "我的电脑\\A17031611.lvlib\\设备状态2"(i16 200 ("设备状态控制字")) -> ()  [unwired: 1 in, 1 out]
                  }
                }
                n360 = local write "STEP2"(w610) -> ()
              }
            }
            n361 = case shown="\"初始化\"" "STEP1" {
              frame "等待", Default {
                n362 = local write "STEP1"("自动" ("STEP1")) -> ()
                n363 = Wait (ms)(milliseconds to wait=u32 200 ("等待时间（毫秒）")) -> ()  [unwired: 1 out]
              }
              frame "初始化" {
                n364 = local write "STEP1"("步骤" ("STEP")) -> ()
                n365 = local write "控制器支架"(T1."控制器支架螺栓1" ("控制器支架")) -> ()
              }
              frame "自动" {
                # "5=31\n4=32\n3=33\n2=34\n1=35"
                n366 = shared-variable "我的电脑\\A17031611.lvlib\\控制器支架螺栓数量"() -> (w58:i16)  [unwired: 1 in, 1 out]
                n367 = shared-variable "我的电脑\\A17031611.lvlib\\设备状态1"() -> (w59:i16)  [unwired: 1 in, 1 out]
                n368 = global read "A170316-11.vi" "控制器支架LED"() -> (w60:refnum<vi>[])
                n369 = case shown="91" w59 {
                  tunnel: w60 -> [_ _ _ _ _ _ _ _ _ _ _ _ _ w104 _ w114 w122 w137]
                  tunnel: w58 -> [_ _ _ _ _ _ _ _ _ _ _ _ _ _ _ _ _ _]
                  frame 0, Default {
                  }
                  frame 10 {
                    n370 = local write "STEP1"("初始化" ("STEP1")) -> ()
                  }
                  frame 30 {
                    n371 = control-ref of="控制器支架螺栓1拧紧确认"() -> (w62:refnum<vi>)
                    n372 = call "Colour.vi"("result"="等待", "colourRef"=w62) -> ()  [unwired: 9 in, 1 out]
                  }
                  frame 31 {
                    n373 = stacked-sequence {
                      frame #0 {
                        n374 = local read "控制器支架"() -> (w64:T1)
                        n375 = control-ref of="控制器支架螺栓1拧紧确认"() -> (w67:refnum<vi>)
                        n376 = Increment(x=w64) -> (x+1=w65:T1)
                        n377 = local write "控制器支架"(w65) -> ()
                        n378 = call "Colour.vi"("result"="OK", "colourRef"=w67) -> ()  [unwired: 9 in, 1 out]
                      }
                      frame #1 {
                        n379 = Wait (ms)(milliseconds to wait=u32 50 ("等待时间（毫秒）")) -> ()  [unwired: 1 out]
                      }
                      frame #2 {
                        n380 = local write "STEP1"("步骤" ("STEP1")) -> ()
                      }
                    }
                  }
                  frame 32 {
                    n381 = control-ref of="控制器支架螺栓2拧紧确认"() -> (w70:refnum<vi>)
                    n382 = call "Colour.vi"("result"="等待", "colourRef"=w70) -> ()  [unwired: 9 in, 1 out]
                  }
                  frame 33 {
                    n383 = stacked-sequence {
                      frame #0 {
                        n384 = local read "控制器支架"() -> (w72:T1)
                        n385 = control-ref of="控制器支架螺栓2拧紧确认"() -> (w74:refnum<vi>)
                        n386 = Increment(x=w72) -> (x+1=w73:T1)
                        n387 = local write "控制器支架"(w73) -> ()
                        n388 = call "Colour.vi"("result"="OK", "colourRef"=w74) -> ()  [unwired: 9 in, 1 out]
                      }
                      frame #1 {
                        n389 = Wait (ms)(milliseconds to wait=u32 50 ("等待时间（毫秒）")) -> ()  [unwired: 1 out]
                      }
                      frame #2 {
                        n390 = local write "STEP1"("步骤" ("STEP1")) -> ()
                      }
                    }
                  }
                  frame 34 {
                    # "控制器支架螺栓1"
                    n391 = control-ref of="控制器支架螺栓3拧紧确认"() -> (w78:refnum<vi>)
                    n392 = call "Colour.vi"("result"="等待", "colourRef"=w78) -> ()  [unwired: 9 in, 1 out]
                  }
                  frame 35 {
                    n393 = stacked-sequence {
                      frame #0 {
                        n394 = control-ref of="控制器支架螺栓3拧紧确认"() -> (w82:refnum<vi>)
                        n395 = local read "控制器支架"() -> (w80:T1)
                        n396 = call "Colour.vi"("result"="OK", "colourRef"=w82) -> ()  [unwired: 9 in, 1 out]
                        n397 = Increment(x=w80) -> (x+1=w81:T1)
                        n398 = local write "控制器支架"(w81) -> ()
                      }
                      frame #1 {
                        n399 = Wait (ms)(milliseconds to wait=u32 50 ("等待时间（毫秒）")) -> ()  [unwired: 1 out]
                      }
                      frame #2 {
                        n400 = local write "STEP1"("步骤" ("STEP1")) -> ()
                      }
                    }
                  }
                  frame 36 {
                    n401 = control-ref of="控制器支架螺栓4拧紧确认"() -> (w86:refnum<vi>)
                    n402 = call "Colour.vi"("result"="等待", "colourRef"=w86) -> ()  [unwired: 9 in, 1 out]
                  }
                  frame 37 {
                    n403 = stacked-sequence {
                      frame #0 {
                        n404 = local read "控制器支架"() -> (w88:T1)
                        n405 = control-ref of="控制器支架螺栓4拧紧确认"() -> (w90:refnum<vi>)
                        n406 = Increment(x=w88) -> (x+1=w89:T1)
                        n407 = local write "控制器支架"(w89) -> ()
                        n408 = call "Colour.vi"("result"="OK", "colourRef"=w90) -> ()  [unwired: 9 in, 1 out]
                      }
                      frame #1 {
                        n409 = Wait (ms)(milliseconds to wait=u32 50 ("毫秒计时值")) -> ()  [unwired: 1 out]
                      }
                      frame #2 {
                        n410 = local write "STEP1"("步骤" ("STEP1")) -> ()
                      }
                    }
                  }
                  frame 38 {
                    n411 = control-ref of="控制器支架螺栓5拧紧确认"() -> (w94:refnum<vi>)
                    n412 = call "Colour.vi"("result"="等待", "colourRef"=w94) -> ()  [unwired: 9 in, 1 out]
                  }
                  frame 39 {
                    n413 = stacked-sequence {
                      frame #0 {
                        n414 = local read "控制器支架"() -> (w96:T1)
                        n415 = control-ref of="控制器支架螺栓5拧紧确认"() -> (w98:refnum<vi>)
                        n416 = Increment(x=w96) -> (x+1=w97:T1)
                        n417 = call "Colour.vi"("result"="OK", "colourRef"=w98) -> ()  [unwired: 9 in, 1 out]
                        n418 = local write "控制器支架"(w97) -> ()
                      }
                      frame #1 {
                        n419 = Wait (ms)(milliseconds to wait=u32 50 ("等待时间（毫秒）")) -> ()  [unwired: 1 out]
                      }
                      frame #2 {
                        n420 = local write "STEP1"("步骤" ("STEP1")) -> ()
                      }
                    }
                  }
                  frame 60 {
                    n421 = control-ref of="控制器支架涂色标"() -> (w102:refnum<vi>)
                    n422 = call "Colour.vi"("result"="等待", "colourRef"=w102) -> ()  [unwired: 9 in, 1 out]
                  }
                  frame 61 {
                    n423 = Index Array(array=w104, index #1=4 ("索引")) -> ()  [unwired: 1 in, 2 out]
                    n424 = stacked-sequence {
                      frame #0 {
                        n425 = local read "控制器支架"() -> (w106:T1)
                        n426 = control-ref of="控制器支架涂色标"() -> (w109:refnum<vi>)
                        n427 = Increment(x=w106) -> (x+1=w107:T1)
                        n428 = call "Colour.vi"("result"="OK", "colourRef"=w109) -> ()  [unwired: 9 in, 1 out]
                        n429 = local write "控制器支架"(w107) -> ()
                      }
                      frame #1 {
                        n430 = Wait (ms)(milliseconds to wait=u32 50 ("等待时间（毫秒）")) -> ()  [unwired: 1 out]
                      }
                      frame #2 {
                        n431 = local write "STEP1"("步骤" ("STEP1")) -> ()
                      }
                    }
                  }
                  frame 70 {
                    n432 = control-ref of="控制器支架安装线卡扎带"() -> (w112:refnum<vi>)
                    n433 = call "Colour.vi"("result"="等待", "colourRef"=w112) -> ()  [unwired: 9 in, 1 out]
                  }
                  frame 81 {
                    n434 = Index Array(array=w114, index=6 ("索引")) -> ()  [unwired: 1 out]
                    n435 = stacked-sequence {
                      frame #0 {
                        n436 = local read "控制器支架"() -> (w116:T1)
                        n437 = control-ref of="控制器支架安装线卡扎带"() -> (w119:refnum<vi>)
                        n438 = Increment(x=w116) -> (x+1=w117:T1)
                        n439 = call "Colour.vi"("result"="OK", "colourRef"=w119) -> ()  [unwired: 9 in, 1 out]
                        n440 = local write "控制器支架"(w117) -> ()
                      }
                      frame #1 {
                        n441 = Wait (ms)(milliseconds to wait=u32 50 ("毫秒计时值")) -> ()  [unwired: 1 out]
                      }
                      frame #2 {
                        n442 = local write "STEP1"("步骤" ("STEP1")) -> ()
                      }
                    }
                  }
                  frame 91 {
                    n443 = for {
                      tunnel: w122 -> [w125] mode=indexing
                      n444 = call "Colour.vi"("result"="", "colourRef"=w125) -> ()  [unwired: 9 in, 1 out]
                    }
                    n445 = shared-variable "我的电脑\\A17031611.lvlib\\设备状态1"(i16 8 ("设备状态")) -> ()  [unwired: 1 in, 1 out]
                    n446 = call "浮动通知2.vi"("通知内容"="控制器和支架合装完成！" ("Status")) -> ()  [unwired: 11 in]
                  }
                  frame 999 {
                    n447 = Index Array(array=w137, index #1=0 ("索引")) -> (element #1=w140:refnum<vi>, element #2=w134:refnum<vi>, element #3=w132:refnum<vi>, element #4=w130:refnum<vi>, element #5=w127:refnum<vi>)  [unwired: 4 in]
                    n448 = call "Colour.vi"("result"="", "colourRef"=w127) -> ()  [unwired: 9 in, 1 out]
                    n449 = call "Colour.vi"("result"="", "colourRef"=w134) -> ()  [unwired: 9 in, 1 out]
                    n450 = call "Colour.vi"("result"="", "colourRef"=w132) -> ()  [unwired: 9 in, 1 out]
                    n451 = call "Colour.vi"("result"="", "colourRef"=w130) -> ()  [unwired: 9 in, 1 out]
                    n452 = call "Colour.vi"("result"="NG", "colourRef"=w140) -> ()  [unwired: 9 in, 1 out]
                    n453 = call "浮动通知2.vi"("通知内容"="安装固定螺栓未完成，请重新安装！" ("Status")) -> ()  [unwired: 11 in]
                    n454 = shared-variable "我的电脑\\A17031611.lvlib\\设备状态1"(i16 10 ("设备状态")) -> ()  [unwired: 1 in, 1 out]
                  }
                }
              }
              frame "步骤" {
                n455 = case shown="\"完成\"" "控制器支架" {
                  selector: "控制器支架" -> [w144 _]
                  tunnel: [w143 "等待"] -> w141
                  frame "控制器支架螺栓1", Default {
                    n456 = global read "Global.vi" "控制器支架"() -> (w146:bool[])
                    n457 = Index Array(array=w146, index=w144) -> (element=w145:bool)
                    n458 = case shown="真" w145 {
                      tunnel: w144 -> [_ w151]
                      tunnel: ["步骤" w150] -> w143
                      frame False {
                        n459 = local read "控制器支架"() -> (w149:T1)
                        n460 = Increment(x=w149) -> (x+1=w148:T1)
                        n461 = local write "控制器支架"(w148) -> ()
                      }
                      frame True {
                        n462 = case shown="\"安装线卡轧带\"" w151 {
                          tunnel: ["等待" "等待" "等待" "等待" "等待" "等待" "等待"] -> w150
                          frame "控制器支架螺栓1", Default {
                            n463 = shared-variable "我的电脑\\A17031611.lvlib\\设备状态1"(i16 30 ("设备状态1")) -> ()  [unwired: 1 in, 1 out]
                          }
                          frame "控制器支架螺栓2" {
                            n464 = shared-variable "我的电脑\\A17031611.lvlib\\设备状态1"(i16 32 ("设备状态1")) -> ()  [unwired: 1 in, 1 out]
                          }
                          frame "控制器支架螺栓3" {
                            n465 = shared-variable "我的电脑\\A17031611.lvlib\\设备状态1"(i16 34 ("设备状态1")) -> ()  [unwired: 1 in, 1 out]
                          }
                          frame "控制器支架螺栓4" {
                            n466 = shared-variable "我的电脑\\A17031611.lvlib\\设备状态1"(i16 36 ("设备状态1")) -> ()  [unwired: 1 in, 1 out]
                          }
                          frame "控制器支架螺栓5" {
                            n467 = shared-variable "我的电脑\\A17031611.lvlib\\设备状态1"(i16 38 ("设备状态1")) -> ()  [unwired: 1 in, 1 out]
                          }
                          frame "涂色标" {
                            n468 = shared-variable "我的电脑\\A17031611.lvlib\\设备状态1"(i16 60 ("设备状态1")) -> ()  [unwired: 1 in, 1 out]
                          }
                          frame "安装线卡轧带" {
                            n469 = shared-variable "我的电脑\\A17031611.lvlib\\设备状态1"(i16 70 ("设备状态1")) -> ()  [unwired: 1 in, 1 out]
                          }
                        }
                      }
                    }
                  }
                  frame "完成" {
                    n470 = shared-variable "我的电脑\\A17031611.lvlib\\设备状态1"(i16 91 ("设备状态")) -> ()  [unwired: 1 in, 1 out]
                  }
                }
                n471 = local write "STEP1"(w141) -> ()
              }
            }
            n472 = global read "Global.vi" "程序关闭"() -> (w53:bool)
          }
        }
        frame Enabled {
        }
      }
      n473 = while {
        stop <- w644 stop-if-true
        n474 = case shown="\"扫电机码\"" "STEP3" {
          frame "等待", Default {
            n475 = local write "STEP3"("自动" ("STEP")) -> ()
            n476 = Wait (ms)(milliseconds to wait=u32 100 ("等待时间（毫秒）")) -> ()  [unwired: 1 out]
          }
          frame "手动" {
            n477 = global read "Global.vi" "ECU自动"() -> (w650:refnum<vi>)
            n478 = shared-variable "我的电脑\\A17031611.lvlib\\设备状态1"(u16 0 ("设备状态")) -> ()  [unwired: 1 in, 1 out]
            n479 = shared-variable "我的电脑\\A17031611.lvlib\\设备状态2"(u16 0 ("设备状态")) -> ()  [unwired: 1 in, 1 out]
            n480 = property class="Bool (严格)"(reference=w650, "Value"=FALSE) -> ()  [unwired: 1 in, 2 out]
            n481 = global read "Global.vi" "电机程序自动"() -> (w653:refnum<vi>)
            n482 = shared-variable "我的电脑\\A17031611.lvlib\\设备状态3"(u16 0 ("设备状态")) -> ()  [unwired: 1 in, 1 out]
            n483 = property class="Bool"(reference=w653, "Value"=FALSE) -> ()  [unwired: 1 in, 2 out]
            n484 = local write "STEP3"("等待" ("STEP")) -> ()
            n485 = Wait (ms)(milliseconds to wait=u32 100 ("等待时间（毫秒）")) -> ()  [unwired: 1 out]
          }
          frame "初始化" {
            n486 = stacked-sequence {
              frame #0 {
                w665 = enum16{"录入", "清空"}."清空" ("功能")
                n487 = global read "Global.vi" "电机生产数量"() -> (w658:refnum<vi>)
                n488 = shared-variable "我的电脑\\Global.lvlib\\工位追溯码"("" ("传感器码")) -> ()  [unwired: 1 in, 1 out]
                n489 = call "物料信息录入.vi"("功能"=w665) -> ("错误输出"=w664:errorcluster)  [unwired: 14 in]
                n490 = call "质量信息录入.vi"("功能"=w665, "错误输入（无错误）"=w664) -> ("错误输出"=w666:errorcluster)  [unwired: 13 in]
                n491 = property class="Num"(reference=w658, "Value"=0 ("磨合次数")) -> ()  [unwired: 1 in, 2 out]
                n492 = call "不合格信息录入.vi"("功能"=w665, "错误输入（无错误）"=w666) -> ()  [unwired: 13 in, 1 out]
                n493 = global read "Global.vi" "电机程序自动"() -> (w662:refnum<vi>)
                n494 = global read "Global.vi" "检测结果"() -> (w660:refnum<vi>)
                n495 = shared-variable "我的电脑\\A17031611.lvlib\\设备状态3"(i16 6 ("设备状态")) -> ()  [unwired: 1 in, 1 out]
                n496 = property class="Bool"(reference=w662, "Value"=TRUE) -> ()  [unwired: 1 in, 2 out]
                n497 = call "Colour.vi"("result"="", "colourRef"=w660) -> ()  [unwired: 9 in, 1 out]
              }
              frame #1 {
                n498 = for {
                  N: 2 -> [_]
                  tunnel: [cluster{dbl[], dbl[]} {[], []}] -> _ mode=indexing
                }
              }
              frame #2 {
                n499 = global read "Global.vi" "Result"() -> (w671:refnum<vi>)
                n500 = property class="Tbl"(reference=w671, "Value"=string[][] []) -> (reference out=w672:refnum<vi>, error out=w673:errorcluster)  [unwired: 1 in]
                n501 = property class="Tbl"(reference=w672, error in=w673, "Row Headers[]"=string[] ["正向空载扭矩最大值", "正向空载扭矩最小值", "正向空载扭矩平均值", "正向空载扭矩波动值", "逆向空载扭矩最大值", "逆向空载扭矩最小值", "逆向空载扭矩平均值", "逆向空载扭矩波动值", "啮合间隙"] ("列首字符串[]")) -> ()  [unwired: 2 out]
              }
              frame #3 {
                n502 = local write "电机步骤"(T3."安装弹簧" ("电机步骤")) -> ()
                n503 = local write "STEP3"("等待" ("STEP")) -> ()
              }
            }
          }
          frame "批次数量判断" {
            n504 = shared-variable "我的电脑\\Global.lvlib\\产品型号"() -> (w681:string, error out=w684:errorcluster)  [unwired: 1 in]
            n505 = global read "Global.vi" "批次"() -> (w682:refnum<vi>)
            n506 = call "获取批次信息.vi"("error in (no error)"=w684, "产品型号"=w681, "Tbl引用句柄"=w682) -> ("error out"=w683:errorcluster)  [unwired: 7 in, 1 out]
            n507 = property class="Tbl"(reference=w682, error in=w683) -> ("Value"=w685:string[][])  [unwired: 2 out]
            n508 = for {
              tunnel: w685 -> [w691] mode=indexing
              tunnel: [w686] -> w680 mode=indexing
              n509 = Index Array(array=w691) -> (element #1=w687:string, element #3=w690:string)  [unwired: 3 in, 1 out]
              n510 = Decimal String To Number(string=w690) -> (number=w689:i32)  [unwired: 2 in, 1 out]
              n511 = Less Or Equal To 0?(x=w689) -> (x <= 0?=w688:bool)
              n512 = case shown="真" w688 {
                tunnel: w687 -> [_ w696]
                tunnel: [TRUE FALSE] -> w686
                frame False {
                }
                frame True {
                  n513 = Concatenate Strings(w696, "数量不足！" ("字符串")) -> (w694:string)
                  n514 = One Button Dialog(message=w694) -> ()  [unwired: 1 in, 1 out]
                }
              }
            }
            n515 = And Array Elements(Boolean array=w680) -> (logical AND=w679:bool)
            n516 = Select(t="扫码" ("STEP"), s=w679, f="手动" ("STEP")) -> (s? t:f=w676:string)
            n517 = local write "STEP3"(w676) -> ()
          }
          frame "扫管柱码" {
            n518 = stacked-sequence {
              frame #0 {
                (unwired) "SELECT\ndbo.[Code].CODE_ID,\ndbo.[Code].CODE_MAIN,\ndbo.[Code].PRODUCT_ID\n\nFROM\ndbo.[Code].CODE_MAIN = 'MACAU3001'" ("格式字符串")
                (unwired) "SELECT\n*\nFROM\ndbo.[Code]\nWHERE\ndbo.[Code].CODE_MAIN = 'MACAU3001'" ("格式字符串")
                (unwired) "UPDATE\ndbo.[Code]\nSET dbo.[Code].CODE_SENSOR = 'henglong'\nWHERE\ndbo.[Code].CODE_MAIN = 'MACAU3001'\n" ("格式字符串")
                w697 = "请扫电机工位主码！" ("提示信息")
                n519 = global read "Global1.vi" "联机模式"() -> (w699:enum16{"单机", "联网"})
                n520 = call "输入框.vi"("提示信息"=w697) -> ("条形码输出"=w698:string)
                n521 = global write "Global1.vi" "电机工位追溯码"(w698) -> ()
                n522 = shared-variable "我的电脑\\Global.lvlib\\工位追溯码"(w698) -> ()  [unwired: 1 in, 1 out]
                n523 = call "浮动通知.vi"("通知内容"=w697) -> ()  [unwired: 11 in]
                n524 = case shown="\"\", 默认" w698 {
                  selector: w698 -> [w703 _]
                  tunnel: [w702 "手动"] -> w700
                  tunnel: w699 -> [w701 _]
                  frame "", Default {
                    n525 = Wait (ms)(milliseconds to wait=u32 50 ("等待时间（毫秒）")) -> ()  [unwired: 1 out]
                    n526 = case shown="\"联网\"" w701 {
                      tunnel: w703 -> [_ w714]
                      tunnel: ["步骤" ("State(s) in Front (\"\")") w713] -> w702
                      frame "单机", Default {
                        n527 = global read "Global.vi" "电机生产数量"() -> (w707:refnum<vi>)
                        n528 = property class="Num"(reference=w707) -> (reference out=w705:refnum<vi>, error out=w709:errorcluster, "Value"=w710:variant)  [unwired: 1 in]
                        n529 = Variant To Data(type=u32 0, Variant=w710) -> (data=w711:u32)  [unwired: 1 in, 1 out]
                        n530 = Increment(x=w711) -> (x+1=w712:u32)
                        n531 = property class="Num"(reference=w705, error in=w709, "Value"=w712) -> ()  [unwired: 2 out]
                      }
                      frame "联网" {
                        n532 = stacked-sequence {
                          tunnel: w714 -> [w721 _ _ _]
                          tunnel: [_ _ _ w743] -> w713
                          frame #0 {
                            n533 = global read "Global1.vi" "PRODUCT_ID"() -> (w718:string)
                            n534 = Format Into String(format string="SELECT\ndbo.[Code].CODE_ID\nFROM\ndbo.[Code]\nWHERE\ndbo.[Code].CODE_MAIN = '%s'\nAND\ndbo.[Code].PRODUCT_ID = %s\n" ("格式字符串"), w721, w718) -> (resulting string=w720:string)  [unwired: 2 in, 1 out]
                            n535 = call "SQL_query.vi"("SQL query"=w720, "联机模式"=enum16{"单机", "联网"}."联网") -> ("data"=w724:string[][])  [unwired: 1 in, 2 out]
                            n536 = Index Array(array=w724, index (row)=0 ("索引 (行)")) -> (element=w723:string[])  [unwired: 1 in]
                            n537 = Index Array(array=w723, index=0 ("索引")) -> (element=w715:string)
                            n538 = global write "Global1.vi" "CODE_ID"(w715) -> ()
                          }
                          frame #1 {
                            n539 = global read "Global1.vi" "前序DEVICE_ID"() -> (w725:string)
                            n540 = global read "Global1.vi" "CODE_ID"() -> (w726:string)
                            n541 = Format Into String(format string="SELECT\ndbo.[Result].RESULT_VALUE\nFROM\ndbo.[Result]\nWHERE\ndbo.[Result].DEVICE_ID = '%s'\nAND\ndbo.[Result].CODE_ID = %s\n" ("格式字符串"), w725, w726) -> (resulting string=w731:string)  [unwired: 2 in, 1 out]
                            n542 = call "SQL_query.vi"("SQL query"=w731, "联机模式"=enum16{"单机", "联网"}."联网") -> ("data"=w734:string[][])  [unwired: 1 in, 2 out]
                            n543 = Index Array(array=w734, index (row)=0 ("索引 (行)")) -> (element=w733:string[])  [unwired: 1 in]
                            n544 = Index Array(array=w733, index=0 ("索引")) -> (element=w727:string)
                            n545 = local write "前序OK？"(w727) -> ()
                          }
                          frame #2 {
                            n546 = disable-structure shown="禁用" {
                              frame Disabled {
                                n547 = global read "Global1.vi" "CODE_ID"() -> (w736:string)
                                n548 = Format Into String(format string="SELECT\ndbo.[Result].RESULT_VALUE\nFROM\ndbo.[Result]\nWHERE\ndbo.[Result].CODE_ID = '%s''" ("格式字符串"), w736) -> (resulting string=w738:string)  [unwired: 2 in, 1 out]
                                n549 = call "SQL_query.vi"("SQL query"=w738, "联机模式"=enum16{"单机", "联网"}."联网") -> ("data"=w741:string[][])  [unwired: 1 in, 2 out]
                                n550 = Index Array(array=w741) -> (element=w739:string[])  [unwired: 2 in]
                                n551 = Index Array(array=w739) -> (element=w740:string)  [unwired: 1 in]
                                n552 = global write "Global1.vi" "RESULT_VALUE"(w740) -> ()
                              }
                              frame Enabled {
                              }
                            }
                          }
                          frame #3 {
                            n553 = local read "前序OK？"() -> (w742:string)
                            n554 = case shown="\"OK\"" w742 {
                              tunnel: ["等待" "等待" "步骤"] -> w743
                              frame Default {
                                (unwired) i16 6 ("设备状态控制字")
                                n555 = global read "Global1.vi" "电机上序状态"() -> (w747:refnum<vi>)
                                n556 = call "浮动通知.vi"("通知内容"="上序漏序！！" ("Status")) -> ()  [unwired: 11 in]
                                n557 = global read "Global.vi" "电机前序显示字"() -> (w745:refnum<vi>)
                                n558 = call "Colour.vi"("result"="等待", "colourRef"=w747) -> ()  [unwired: 9 in, 1 out]
                                n559 = Wait (ms)(milliseconds to wait=u32 2000 ("等待时间（毫秒）")) -> ()  [unwired: 1 out]
                                n560 = property class="Str"(reference=w745, "Value"="漏序 " ("值")) -> ()  [unwired: 1 in, 2 out]
                              }
                              frame "NG" {
                                (unwired) i16 6 ("设备状态控制字")
                                n561 = global read "Global1.vi" "电机上序状态"() -> (w754:refnum<vi>)
                                n562 = call "浮动通知.vi"("通知内容"="上序生产结果不合格！" ("Status")) -> ()  [unwired: 11 in]
                                n563 = global read "Global.vi" "电机前序显示字"() -> (w752:refnum<vi>)
                                n564 = call "Colour.vi"("result"="NG", "colourRef"=w754) -> ()  [unwired: 9 in, 1 out]
                                n565 = Wait (ms)(milliseconds to wait=u32 2000 ("等待时间（毫秒）")) -> ()  [unwired: 1 out]
                                n566 = property class="Str"(reference=w752, "Value"="NG " ("值")) -> ()  [unwired: 1 in, 2 out]
                              }
                              frame "OK" {
                                n567 = global read "Global.vi" "电机生产数量"() -> (w768:refnum<vi>)
                                n568 = global read "Global1.vi" "电机上序状态"() -> (w761:refnum<vi>)
                                n569 = property class="Num"(reference=w768) -> (reference out=w769:refnum<vi>, error out=w767:errorcluster, "Value"=w766:variant)  [unwired: 1 in]
                                n570 = global read "Global.vi" "电机前序显示字"() -> (w759:refnum<vi>)
                                n571 = call "Colour.vi"("result"="OK", "colourRef"=w761) -> ()  [unwired: 9 in, 1 out]
                                n572 = Variant To Data(type=u32 0, Variant=w766) -> (data=w765:u32)  [unwired: 1 in, 1 out]
                                n573 = Increment(x=w765) -> (x+1=w764:u32)
                                n574 = property class="Num"(reference=w769, error in=w767, "Value"=w764) -> ()  [unwired: 2 out]
                                n575 = property class="Str"(reference=w759, "Value"="OK" ("值")) -> ()  [unwired: 1 in, 2 out]
                              }
                            }
                          }
                        }
                      }
                    }
                  }
                  frame "exit" {
                  }
                }
                n576 = local write "STEP3"(w700) -> ()
              }
              frame #1 {
                n577 = Wait (ms)(milliseconds to wait=u32 100 ("等待时间（毫秒）")) -> ()  [unwired: 1 out]
              }
            }
          }
          frame "扫电机码" {
            n578 = stacked-sequence {
              frame #0 {
                w772 = "请扫电机码！" ("提示信息")
                n579 = call "输入框.vi"("提示信息"=w772) -> ("条形码输出"=w773:string)
                n580 = call "浮动通知.vi"("通知内容"=w772) -> ()  [unwired: 11 in]
                n581 = case shown="\"\", 默认" w773 {
                  selector: w773 -> [w775 _]
                  tunnel: [w776 "手动"] -> w774
                  frame "", Default {
                    n582 = global read "Global1.vi" "联机模式"() -> (w777:enum16{"单机", "联网"})
                    n583 = shared-variable "我的电脑\\Global.lvlib\\电机码"(w775) -> ()  [unwired: 1 in, 1 out]
                    n584 = global write "Global1.vi" "电机码"(w775) -> ()
                    n585 = case shown="\"联网\"" w777 {
                      tunnel: w775 -> [_ _]
                      tunnel: ["步骤" ("State(s) in Front (\"\")") "步骤" ("State(s) in Front (\"\")")] -> w776
                      frame "单机", Default {
                      }
                      frame "联网" {
                        n586 = disable-structure shown="禁用" {
                          frame Disabled {
                            n587 = shared-variable "我的电脑\\A17031611.lvlib\\电机安装螺栓数量"() -> (w780:i16)  [unwired: 1 in, 1 out]
                            n588 = case shown="2, 默认" w780 {
                              frame 2, Default {
                                n589 = shared-variable "我的电脑\\A17031611.lvlib\\设备状态3"(i16 41 ("设备状态控制字")) -> ()  [unwired: 1 in, 1 out]
                              }
                              frame 3 {
                                n590 = shared-variable "我的电脑\\A17031611.lvlib\\设备状态3"(i16 40 ("设备状态控制字")) -> ()  [unwired: 1 in, 1 out]
                              }
                            }
                          }
                          frame Enabled {
                          }
                        }
                      }
                    }
                  }
                  frame "exit" {
                  }
                }
                n591 = local write "STEP3"(w774) -> ()
              }
              frame #1 {
                n592 = Wait (ms)(milliseconds to wait=u32 100 ("等待时间（毫秒）")) -> ()  [unwired: 1 out]
              }
            }
          }
          frame "录入批次" {
            n593 = shared-variable "我的电脑\\Global.lvlib\\产品型号"() -> (w786:string)  [unwired: 1 in, 1 out]
            n594 = call "更新批次.vi"("型号"=w786) -> ("error out"=w787:errorcluster)  [unwired: 10 in]
            n595 = call "更新易损件.vi"("error in (no error)"=w787) -> ("error out"=w790:errorcluster)  [unwired: 10 in]
            n596 = global read "Global.vi" "批次"() -> (w788:refnum<vi>)
            n597 = property class="Tbl"(reference=w788, error in=w790) -> ("Value"=w789:string[][])  [unwired: 2 out]
            n598 = for {
              tunnel: w789 -> [w793] mode=indexing
              n599 = Index Array(array=w793) -> (element #1=w792:string, element #2=w791:string)  [unwired: 2 in]
              n600 = call "物料信息录入.vi"("物料名称"=w792, "功能"=enum16{"录入", "清空"}."录入", "物料编码"=w791) -> ()  [unwired: 12 in, 1 out]
            }
            n601 = local write "STEP3"("等待" ("STEP")) -> ()
          }
          frame "自动" {
            n602 = shared-variable "我的电脑\\A17031611.lvlib\\电机安装螺栓数量"() -> (w795:i16)  [unwired: 1 in, 1 out]
            n603 = shared-variable "我的电脑\\A17031611.lvlib\\设备状态3"() -> (w796:i16)  [unwired: 1 in, 1 out]
            n604 = global read "A170316-11.vi" "电机安装LED"() -> (w797:refnum<vi>[])
            n605 = case shown="0" w796 {
              tunnel: w795 -> [_ _ _ _ _ _ _ _ _ _ _ _ _ _ _ w849 w860 _ _ _ _ _ _ w913 w925 _ _ _ _ _ _ _ _ _ _ _ _ _ _ _]
              tunnel: w797 -> [_ _ _ _ w803 _ _ _ _ _ _ _ _ w838 _ w851 w859 _ _ _ _ _ _ w912 w924 _ _ _ _ _ w956 w959 _ _ w1000 _ _ _ _ _]
              frame -128 {
                n606 = call "浮动通知.vi"("通知内容"="复位中……" ("Status")) -> ()  [unwired: 11 in]
                n607 = global read "Global.vi" "电机程序自动"() -> (w799:refnum<vi>)
                n608 = property class="Bool"(reference=w799, "Value"=FALSE) -> ()  [unwired: 1 in, 2 out]
              }
              frame 0 {
              }
              frame 5 {
                n609 = call "浮动通知.vi"("通知内容"="复位完成" ("Status")) -> ()  [unwired: 11 in]
              }
              frame 6 {
                n610 = call "浮动通知.vi"("通知内容"="请按启动扫电机工位主码") -> ()  [unwired: 11 in]
              }
              frame 7 {
                n611 = for {
                  tunnel: w803 -> [w811] mode=indexing
                  n612 = call "Colour -电机.vi"("result"="", "colourRef"=w811) -> ()  [unwired: 9 in, 1 out]
                }
                n613 = global read "Global.vi" "电机结果显示"() -> (w807:refnum<vi>)
                n614 = shared-variable "我的电脑\\Global.lvlib\\工位追溯码"("" ("传感器码")) -> ()  [unwired: 1 in, 1 out]
                n615 = property class="Str"(reference=w807, "Value"="..." ("结果显示")) -> (reference out=w806:refnum<vi>)  [unwired: 1 in, 1 out]
                n616 = property class="Str"(reference=w806, "Text.TextColor"=u32 16776960) -> ()  [unwired: 1 in, 2 out]
                n617 = local write "STEP3"("扫管柱码" ("STEP3")) -> ()
              }
              frame 8 {
                n618 = call "浮动通知.vi"("通知内容"="程序停止！" ("Status")) -> ()  [unwired: 11 in]
              }
              frame 9 {
                n619 = call "浮动通知.vi"("通知内容"="套花键中" ("Status")) -> ()  [unwired: 11 in]
              }
              frame 10 {
                n620 = local write "STEP3"("步骤" ("STEP3")) -> ()
                n621 = call "浮动通知.vi"("通知内容"="请安装胶垫弹簧并拍照确认！" ("Status")) -> ()  [unwired: 11 in]
              }
              frame 16 {
                n622 = control-ref of="请拾取弹簧"() -> (w817:refnum<vi>)
                n623 = call "Colour -电机.vi"("result"="等待", "colourRef"=w817) -> ()  [unwired: 9 in, 1 out]
                n624 = call "浮动通知.vi"("通知内容"="请拾取弹簧并安装到位") -> ()  [unwired: 11 in]
              }
              frame 17 {
                n625 = stacked-sequence {
                  frame #0 {
                    n626 = local read "电机步骤"() -> (w820:T3)
                    n627 = control-ref of="请拾取弹簧"() -> (w821:refnum<vi>)
                    n628 = Increment(x=w820) -> (x+1=w819:T3)
                    n629 = local write "电机步骤"(w819) -> ()
                    n630 = call "Colour -电机.vi"("result"="OK", "colourRef"=w821) -> ()  [unwired: 9 in, 1 out]
                  }
                  frame #1 {
                    n631 = Wait (ms)(milliseconds to wait=u32 100 ("等待时间（毫秒）")) -> ()  [unwired: 1 out]
                  }
                  frame #2 {
                    n632 = local write "STEP3"("扫电机码" ("STEP3")) -> ()
                  }
                }
              }
              frame 18 {
                n633 = control-ref of="请拾取O型圈"() -> (w826:refnum<vi>)
                n634 = call "浮动通知.vi"("通知内容"="请拾O型圈") -> ()  [unwired: 11 in]
                n635 = call "Colour -电机.vi"("result"="等待", "colourRef"=w826) -> ()  [unwired: 9 in, 1 out]
              }
              frame 19 {
                n636 = stacked-sequence {
                  frame #0 {
                    n637 = local read "电机步骤"() -> (w829:T3)
                    n638 = control-ref of="请拾取O型圈"() -> (w830:refnum<vi>)
                    n639 = Increment(x=w829) -> (x+1=w828:T3)
                    n640 = local write "电机步骤"(w828) -> ()
                    n641 = call "Colour -电机.vi"("result"="OK", "colourRef"=w830) -> ()  [unwired: 9 in, 1 out]
                  }
                  frame #1 {
                    n642 = Wait (ms)(milliseconds to wait=u32 100 ("等待时间（毫秒）")) -> ()  [unwired: 1 out]
                  }
                  frame #2 {
                    n643 = local write "STEP3"("步骤" ("STEP3")) -> ()
                  }
                }
              }
              frame 20 {
                n644 = control-ref of="安装弹性垫圈弹簧并按启动拍照"() -> (w835:refnum<vi>)
                n645 = call "Colour -电机.vi"("result"="等待", "colourRef"=w835) -> ()  [unwired: 9 in, 1 out]
                n646 = call "浮动通知.vi"("通知内容"="请安装胶垫弹簧并拍照确认！" ("Status")) -> ()  [unwired: 11 in]
              }
              frame 30 {
                n647 = Index Array(array=w838, index #1=0 ("索引")) -> ()  [unwired: 1 in, 2 out]
                n648 = control-ref of="安装弹性垫圈弹簧并按启动拍照"() -> (w837:refnum<vi>)
                n649 = call "Colour.vi"("result"="NG", "colourRef"=w837) -> ()  [unwired: 9 in, 1 out]
                n650 = call "浮动通知.vi"("通知内容"="请安装胶垫弹簧并拍照确认！" ("Status")) -> ()  [unwired: 11 in]
              }
              frame 31 {
                n651 = stacked-sequence {
                  frame #0 {
                    n652 = local read "电机步骤"() -> (w843:T3)
                    n653 = control-ref of="安装弹性垫圈弹簧并按启动拍照"() -> (w845:refnum<vi>)
                    n654 = Increment(x=w843) -> (x+1=w842:T3)
                    n655 = call "Colour -电机.vi"("result"="OK", "colourRef"=w845) -> ()  [unwired: 9 in, 1 out]
                    n656 = local write "电机步骤"(w842) -> ()
                    n657 = call "浮动通知.vi"("通知内容"="请扫电机码！" ("Status")) -> ()  [unwired: 11 in]
                  }
                  frame #1 {
                    n658 = Wait (ms)(milliseconds to wait=u32 10 ("等待时间（毫秒）")) -> ()  [unwired: 1 out]
                  }
                  frame #2 {
                    n659 = local write "STEP3"("扫电机码" ("STEP3")) -> ()
                  }
                }
              }
              frame 35 {
                n660 = case shown="2" w849 {
                  tunnel: w851 -> [_ w857]
                  frame 0, Default {
                  }
                  frame 2 {
                    n661 = Index Array(array=w857, index #1=0 ("索引")) -> (element #1=w855:refnum<vi>, element #2=w853:refnum<vi>)  [unwired: 1 in]
                    n662 = call "Colour -电机.vi"("result"="OK", "colourRef"=w855) -> ()  [unwired: 9 in, 1 out]
                    n663 = call "Colour -电机.vi"("result"="等待", "colourRef"=w853) -> ()  [unwired: 9 in, 1 out]
                    n664 = shared-variable "我的电脑\\A17031611.lvlib\\设备状态3"(i16 41 ("设备状态")) -> ()  [unwired: 1 in, 1 out]
                  }
                }
                n665 = call "浮动通知.vi"("通知内容"="请安装固定螺栓1并确认扭矩！" ("Status")) -> ()  [unwired: 11 in]
              }
              frame 36 {
                n666 = case shown="2" w860 {
                  tunnel: w859 -> [w862 w875 w879]
                  frame 1 {
                    n667 = Index Array(array=w862, index=1 ("索引")) -> (element=w869:refnum<vi>)
                    n668 = Index Array(array=w862, index=4 ("索引")) -> (element=w863:refnum<vi>)
                    n669 = call "Colour.vi"("result"="OK", "colourRef"=w869) -> ()  [unwired: 9 in, 1 out]
                    n670 = call "Colour.vi"("result"="等待", "colourRef"=w863) -> ()  [unwired: 9 in, 1 out]
                    n671 = call "浮动通知.vi"("通知内容"="请按启动拍照确认电机方向！" ("Status")) -> ()  [unwired: 11 in]
                    n672 = shared-variable "我的电脑\\A17031611.lvlib\\设备状态1"(i16 70 ("设备状态")) -> ()  [unwired: 1 in, 1 out]
                  }
                  frame 2 {
                    n673 = Index Array(array=w875, index #1=0 ("索引")) -> (element #1=w873:refnum<vi>, element #2=w871:refnum<vi>)  [unwired: 2 in, 1 out]
                    n674 = call "Colour -电机.vi"("result"="OK", "colourRef"=w873) -> ()  [unwired: 9 in, 1 out]
                    n675 = call "Colour -电机.vi"("result"="等待", "colourRef"=w871) -> ()  [unwired: 9 in, 1 out]
                    n676 = call "浮动通知.vi"("通知内容"="请安装固定螺栓1并确认扭矩！" ("Status")) -> ()  [unwired: 11 in]
                  }
                  frame Default {
                    n677 = Index Array(array=w879, index #1=1 ("索引")) -> (element #1=w883:refnum<vi>, element #2=w884:refnum<vi>)  [unwired: 1 in]
                    n678 = call "Colour.vi"("result"="OK", "colourRef"=w883) -> ()  [unwired: 9 in, 1 out]
                    n679 = call "浮动通知.vi"("通知内容"="请安装固定螺栓2并确认扭矩！" ("Status")) -> ()  [unwired: 11 in]
                    n680 = call "Colour.vi"("result"="等待", "colourRef"=w884) -> ()  [unwired: 9 in, 1 out]
                    n681 = shared-variable "我的电脑\\A17031611.lvlib\\设备状态3"(i16 40 ("设备状态")) -> ()  [unwired: 1 in, 1 out]
                  }
                }
              }
              frame 40 {
                n682 = control-ref of="电机安装螺栓1扭矩确认"() -> (w885:refnum<vi>)
                n683 = call "Colour -电机.vi"("result"="等待", "colourRef"=w885) -> ()  [unwired: 9 in, 1 out]
                n684 = call "浮动通知.vi"("通知内容"="请安装固定螺栓1并确认扭矩！" ("Status")) -> ()  [unwired: 11 in]
              }
              frame 41 {
                n685 = stacked-sequence {
                  frame #0 {
                    n686 = local read "电机步骤"() -> (w889:T3)
                    n687 = control-ref of="电机安装螺栓1扭矩确认"() -> (w890:refnum<vi>)
                    n688 = Increment(x=w889) -> (x+1=w888:T3)
                    n689 = local write "电机步骤"(w888) -> ()
                    n690 = call "Colour -电机.vi"("result"="OK", "colourRef"=w890) -> ()  [unwired: 9 in, 1 out]
                  }
                  frame #1 {
                    n691 = Wait (ms)(milliseconds to wait=u32 10 ("等待时间（毫秒）")) -> ()  [unwired: 1 out]
                  }
                  frame #2 {
                    n692 = local write "STEP3"("步骤" ("STEP3")) -> ()
                  }
                }
              }
              frame 42 {
                n693 = control-ref of="电机安装螺栓2扭矩确认"() -> (w895:refnum<vi>)
                n694 = call "浮动通知.vi"("通知内容"="请安装固定螺栓2并确认扭矩！" ("Status")) -> ()  [unwired: 11 in]
                n695 = call "Colour -电机.vi"("result"="等待", "colourRef"=w895) -> ()  [unwired: 9 in, 1 out]
              }
              frame 43 {
                n696 = stacked-sequence {
                  frame #0 {
                    n697 = local read "电机步骤"() -> (w898:T3)
                    n698 = control-ref of="电机安装螺栓2扭矩确认"() -> (w899:refnum<vi>)
                    n699 = Increment(x=w898) -> (x+1=w897:T3)
                    n700 = local write "电机步骤"(w897) -> ()
                    n701 = call "Colour -电机.vi"("result"="OK", "colourRef"=w899) -> ()  [unwired: 9 in, 1 out]
                  }
                  frame #1 {
                    n702 = Wait (ms)(milliseconds to wait=u32 10 ("等待时间（毫秒）")) -> ()  [unwired: 1 out]
                  }
                  frame #2 {
                    n703 = local write "STEP3"("步骤" ("STEP3")) -> ()
                  }
                }
              }
              frame 44 {
                n704 = control-ref of="电机安装螺栓3扭矩确认"() -> (w904:refnum<vi>)
                n705 = call "浮动通知.vi"("通知内容"="请安装固定螺栓3并确认扭矩！" ("Status")) -> ()  [unwired: 11 in]
                n706 = call "Colour -电机.vi"("result"="等待", "colourRef"=w904) -> ()  [unwired: 9 in, 1 out]
              }
              frame 45 {
                n707 = stacked-sequence {
                  frame #0 {
                    n708 = local read "电机步骤"() -> (w906:T3)
                    n709 = control-ref of="电机安装螺栓3扭矩确认"() -> (w908:refnum<vi>)
                    n710 = Increment(x=w906) -> (x+1=w907:T3)
                    n711 = call "Colour -电机.vi"("result"="OK", "colourRef"=w908) -> ()  [unwired: 9 in, 1 out]
                    n712 = local write "电机步骤"(w907) -> ()
                  }
                  frame #1 {
                    n713 = Wait (ms)(milliseconds to wait=u32 10 ("等待时间（毫秒）")) -> ()  [unwired: 1 out]
                  }
                  frame #2 {
                    n714 = local write "STEP3"("步骤" ("STEP3")) -> ()
                  }
                }
              }
              frame 51 {
                n715 = case shown="2" w913 {
                  tunnel: w912 -> [_ _ w918]
                  frame 0, 1 {
                  }
                  frame 2 {
                    n716 = call "浮动通知.vi"("通知内容"="请按启动按钮拍照确认！" ("Status")) -> ()  [unwired: 11 in]
                    n717 = shared-variable "我的电脑\\A17031611.lvlib\\设备状态3"(i16 70 ("设备状态")) -> ()  [unwired: 1 in, 1 out]
                  }
                  frame Default {
                    n718 = Index Array(array=w918, index #1=2 ("索引")) -> (element #1=w922:refnum<vi>, element #2=w919:refnum<vi>)  [unwired: 1 in]
                    n719 = call "浮动通知.vi"("通知内容"="请按启动按钮拍照确认！" ("Status")) -> ()  [unwired: 11 in]
                    n720 = call "Colour.vi"("result"="OK", "colourRef"=w922) -> ()  [unwired: 9 in, 1 out]
                    n721 = call "Colour.vi"("result"="等待", "colourRef"=w919) -> ()  [unwired: 9 in, 1 out]
                    n722 = shared-variable "我的电脑\\A17031611.lvlib\\设备状态3"(i16 70 ("设备状态")) -> ()  [unwired: 1 in, 1 out]
                  }
                }
              }
              frame 61 {
                n723 = case shown="默认" w925 {
                  tunnel: w924 -> [w930 _]
                  frame Default {
                    n724 = Index Array(array=w930, index #1=3 ("索引")) -> (element #1=w932:refnum<vi>, element #2=w933:refnum<vi>)  [unwired: 1 in]
                    n725 = call "Colour.vi"("result"="OK", "colourRef"=w932) -> ()  [unwired: 9 in, 1 out]
                    n726 = call "Colour.vi"("result"="等待", "colourRef"=w933) -> ()  [unwired: 9 in, 1 out]
                    n727 = call "浮动通知.vi"("通知内容"="请按启动拍照确认！" ("Status")) -> ()  [unwired: 11 in]
                    n728 = shared-variable "我的电脑\\A17031611.lvlib\\设备状态3"(i16 70 ("设备状态")) -> ()  [unwired: 1 in, 1 out]
                  }
                  frame 0..2 {
                  }
                }
              }
              frame 70 {
                n729 = control-ref of="按启动按钮拍照确认"() -> (w935:refnum<vi>)
                n730 = call "浮动通知.vi"("通知内容"="请按启动拍照确认！" ("Status")) -> ()  [unwired: 11 in]
                n731 = call "Colour -电机.vi"("result"="等待", "colourRef"=w935) -> ()  [unwired: 9 in, 1 out]
              }
              frame 80 {
                n732 = control-ref of="按启动按钮拍照确认"() -> (w938:refnum<vi>)
                n733 = call "Colour -电机.vi"("result"="NG", "colourRef"=w938) -> ()  [unwired: 9 in, 1 out]
              }
              frame 81 {
                n734 = stacked-sequence {
                  frame #0 {
                    n735 = local read "电机步骤"() -> (w939:T3)
                    n736 = control-ref of="按启动按钮拍照确认"() -> (w942:refnum<vi>)
                    n737 = Increment(x=w939) -> (x+1=w940:T3)
                    n738 = local write "电机步骤"(w940) -> ()
                    n739 = call "Colour -电机.vi"("result"="OK", "colourRef"=w942) -> ()  [unwired: 9 in, 1 out]
                  }
                  frame #1 {
                    n740 = Wait (ms)(milliseconds to wait=u32 5 ("等待时间（毫秒）")) -> ()  [unwired: 1 out]
                  }
                  frame #2 {
                    n741 = local write "STEP3"("步骤" ("STEP3")) -> ()
                  }
                }
              }
              frame 90 {
                n742 = control-ref of="涂色标"() -> (w946:refnum<vi>)
                n743 = call "浮动通知.vi"("通知内容"="请给固定螺栓涂色标！" ("Status")) -> ()  [unwired: 11 in]
                n744 = call "Colour -电机.vi"("result"="等待", "colourRef"=w946) -> ()  [unwired: 9 in, 1 out]
              }
              frame 91 {
                n745 = stacked-sequence {
                  frame #0 {
                    n746 = local read "电机步骤"() -> (w949:T3)
                    n747 = control-ref of="涂色标"() -> (w950:refnum<vi>)
                    n748 = Increment(x=w949) -> (x+1=w948:T3)
                    n749 = local write "电机步骤"(w948) -> ()
                    n750 = call "Colour -电机.vi"("result"="OK", "colourRef"=w950) -> ()  [unwired: 9 in, 1 out]
                  }
                  frame #1 {
                    n751 = Wait (ms)(milliseconds to wait=u32 10 ("等待时间（毫秒）")) -> ()  [unwired: 1 out]
                  }
                  frame #2 {
                    n752 = local write "STEP3"("步骤" ("STEP3")) -> ()
                  }
                }
              }
              frame 100 {
                n753 = Index Array(array=w956, index #1=4 ("索引")) -> ()  [unwired: 1 in, 2 out]
                n754 = control-ref of="安装扎带并取走工件"() -> (w955:refnum<vi>)
                n755 = call "Colour -电机.vi"("result"="等待", "colourRef"=w955) -> ()  [unwired: 9 in, 1 out]
                n756 = call "浮动通知.vi"("通知内容"="请安装轧带并取走工件" ("Status")) -> ()  [unwired: 11 in]
              }
              frame 101 {
                n757 = Index Array(array=w959, index #1=5 ("索引")) -> ()  [unwired: 1 in, 2 out]
                n758 = stacked-sequence {
                  frame #0 {
                    n759 = local read "电机步骤"() -> (w962:T3)
                    n760 = control-ref of="安装扎带并取走工件"() -> (w963:refnum<vi>)
                    n761 = Increment(x=w962) -> (x+1=w961:T3)
                    n762 = local write "电机步骤"(w961) -> ()
                    n763 = call "Colour -电机.vi"("result"="OK", "colourRef"=w963) -> ()  [unwired: 9 in, 1 out]
                  }
                  frame #1 {
                    n764 = Wait (ms)(milliseconds to wait=u32 100 ("等待时间（毫秒）")) -> ()  [unwired: 1 out]
                  }
                  frame #2 {
                    n765 = local write "STEP3"("步骤" ("STEP3")) -> ()
                  }
                }
              }
              frame 200 {
                n766 = global read "Global1.vi" "联机模式"() -> (w967:enum16{"单机", "联网"})
                n767 = Wait (ms)(milliseconds to wait=u32 100 ("等待时间（毫秒）")) -> ()  [unwired: 1 out]
                n768 = case shown="\"联网\"" w967 {
                  frame "单机", Default {
                    n769 = global read "Global.vi" "检测结果"() -> (w977:refnum<vi>)
                    n770 = call "浮动通知.vi"("通知内容"="产品合格！" ("Status")) -> ()  [unwired: 11 in]
                    n771 = call "Colour.vi"("result"="OK", "colourRef"=w977) -> ()  [unwired: 9 in, 1 out]
                    n772 = global read "Global.vi" "电机结果显示"() -> (w974:refnum<vi>)
                    n773 = local write "电机步骤"(T3."安装弹簧" ("电机步骤")) -> ()
                    n774 = local write "STEP3"("初始化" ("STEP3")) -> ()
                    n775 = property class="Str"(reference=w974, "Value"="OK" ("结果显示")) -> (reference out=w973:refnum<vi>)  [unwired: 1 in, 1 out]
                    n776 = property class="Str"(reference=w973, "Text.TextColor"=u32 6618880) -> ()  [unwired: 1 in, 2 out]
                  }
                  frame "联网" {
                    n777 = global read "Global.vi" "检测结果"() -> (w979:refnum<vi>)
                    n778 = global write "Global1.vi" "电机工位生产结果"("OK" ("电机工位生产结果")) -> ()
                    n779 = call "浮动通知.vi"("通知内容"="产品合格！" ("Status")) -> ()  [unwired: 11 in]
                    n780 = call "Colour -电机.vi"("result"="OK", "colourRef"=w979) -> ()  [unwired: 9 in, 1 out]
                    n781 = global read "Global.vi" "电机结果显示"() -> (w987:refnum<vi>)
                    n782 = property class="Str"(reference=w987, "Value"="OK" ("结果显示")) -> (reference out=w984:refnum<vi>)  [unwired: 1 in, 1 out]
                    n783 = global read "Global1.vi" "联机模式"() -> (w980:enum16{"单机", "联网"})
                    n784 = property class="Str"(reference=w984, "Text.TextColor"=u32 6618880) -> ()  [unwired: 1 in, 2 out]
                    n785 = case shown="\"联网\"" w980 {
                      tunnel: ["自动" "录入数据库" ("STEP3")] -> w981
                      frame "单机", Default {
                        n786 = shared-variable "我的电脑\\A17031611.lvlib\\设备状态3"(i16 6 ("设备状态")) -> ()  [unwired: 1 in, 1 out]
                      }
                      frame "联网" {
                      }
                    }
                    n787 = local write "STEP3"(w981) -> ()
                  }
                }
              }
              frame 201 {
                n788 = global read "Global.vi" "检测结果"() -> (w996:refnum<vi>)
                n789 = call "Colour.vi"("result"="NG", "colourRef"=w996) -> ()  [unwired: 9 in, 1 out]
                n790 = call "浮动通知.vi"("通知内容"="产品不合格！" ("Status")) -> ()  [unwired: 11 in]
                n791 = global read "Global.vi" "电机结果显示"() -> (w995:refnum<vi>)
                n792 = property class="Str"(reference=w995, "Value"="NG" ("结果显示")) -> (reference out=w994:refnum<vi>)  [unwired: 1 in, 1 out]
                n793 = property class="Str"(reference=w994, "Text.TextColor"=u32 16711680) -> ()  [unwired: 1 in, 2 out]
              }
              frame 999 {
                n794 = Index Array(array=w1000, index #1=0 ("索引")) -> (element #1=w1008:refnum<vi>, element #2=w1009:refnum<vi>, element #3=w1001:refnum<vi>, element #4=w998:refnum<vi>)  [unwired: 3 in]
                n795 = call "Colour.vi"("result"="", "colourRef"=w1001) -> ()  [unwired: 9 in, 1 out]
                n796 = call "Colour.vi"("result"="", "colourRef"=w998) -> ()  [unwired: 9 in, 1 out]
                n797 = call "Colour.vi"("result"="NG", "colourRef"=w1009) -> ()  [unwired: 9 in, 1 out]
                n798 = call "Colour.vi"("result"="OK", "colourRef"=w1008) -> ()  [unwired: 9 in, 1 out]
                n799 = call "浮动通知.vi"("通知内容"="请重新安装固定螺栓！" ("Status")) -> ()  [unwired: 11 in]
                n800 = shared-variable "我的电脑\\A17031611.lvlib\\设备状态3"(i16 40 ("设备状态")) -> ()  [unwired: 1 in, 1 out]
              }
              frame 1024 {
                n801 = call "浮动通知.vi"("通知内容"="急停！" ("Status")) -> ()  [unwired: 11 in]
                n802 = global read "Global.vi" "电机程序自动"() -> (w1011:refnum<vi>)
                n803 = property class="Bool"(reference=w1011, "Value"=FALSE) -> ()  [unwired: 1 in, 2 out]
              }
              frame 3721 {
                n804 = local write "STEP3"("不合格锁定" ("STEP")) -> ()
                n805 = call "浮动通知.vi"("通知内容"="产品不合格程序锁定！" ("Status")) -> ()  [unwired: 11 in]
              }
              frame 3722 {
                n806 = global read "Global.vi" "电机程序自动"() -> (w1016:refnum<vi>)
                n807 = call "浮动通知.vi"("通知内容"="授权成功，请复位！" ("Status")) -> ()  [unwired: 11 in]
                n808 = property class="Bool"(reference=w1016, "Value"=FALSE) -> ()  [unwired: 1 in, 2 out]
              }
              frame 3723 {
                n809 = call "浮动通知.vi"("通知内容"="请取出不合格产品并摆放至不合格品区！" ("Status")) -> ()  [unwired: 11 in]
              }
              frame Default {
              }
            }
          }
          frame "录入数据库" {
            n810 = stacked-sequence {
              frame #0 {
                n811 = Get Date/Time String(date format (0)=enum16{"short", "long", "abbreviated"}."short" ("日期格式(0)"), want seconds? (F)=FALSE ("需要秒？(F)")) -> (date string=w1028:string, time string=w1029:string)  [unwired: 1 in]
                n812 = global read "Global1.vi" "电机工位生产结果"() -> (w1023:string)
                n813 = global read "Global1.vi" "DEVICE_ID"() -> (w1032:string)
                n814 = global read "Global1.vi" "USER_ID"() -> (w1030:string)
                n815 = global read "Global1.vi" "CODE_ID"() -> (w1031:string)
                n816 = Concatenate Strings(w1028, " " ("字符串"), w1029) -> (w1024:string)
                n817 = Decimal String To Number(string=w1032, default (0L)=i64 0 ("默认(0 I32)")) -> (number=w1021:i64)  [unwired: 1 in, 1 out]
                n818 = Decimal String To Number(string=w1030, default (0L)=i64 0 ("默认(0 I32)")) -> (number=w1020:i64)  [unwired: 1 in, 1 out]
                n819 = Decimal String To Number(string=w1031, default (0L)=i64 0 ("默认(0 I32)")) -> (number=w1019:i64)  [unwired: 1 in, 1 out]
                n820 = global read "Global1.vi" "联机模式"() -> (w1039:enum16{"单机", "联网"})
                n821 = Search and Replace String(replace all?=TRUE ("替换全部？(F)"), input string=w1024, search string="/" ("替换字符串(\"\")"), replace string="-" ("替换字符串(\"\")")) -> (result string=w1022:string)  [unwired: 4 in, 3 out]
                n822 = Bundle(w1021, w1020, w1019, "电机工位生产结果"=w1023, "result string"=w1022) -> (w1045:T8)  [unwired: 1 in]
                n823 = call "GetSQLstring.vi"("联机模式"=w1039) -> ("错误输出"=w1042:errorcluster, "连接字符串"=w1041:string)  [unwired: 9 in]
                n824 = Build Array(w1045) -> (w1046:T9)
                n825 = call-poly <vilib>:"DB Tools Open Connection.vi"("error in (no error)"=w1042, "connection information"=w1041) -> ("error out"=w1040:errorcluster, "connection reference"=w1043:T6)  [unwired: 6 in]
                n826 = for {
                  tunnel: w1046 -> [w1051] mode=indexing
                  tunnel: w1043 -> [w1049]
                  shift-right: [w1047] -> w1044
                  shift-left: w1040 -> [w1054]
                  w1050 = string[] ["DEVICE_ID", "USER_ID", "CODE_ID", "RESULT_VALUE", "RESULT_TIME"] ("columns")
                  w1052 = "Result" ("table")
                  n827 = call <vilib>:"DB Tools Insert Data.vi"("data"=w1051, "error in (no error)"=w1054, "columns"=w1050, "table"=w1052, "connection reference"=w1049) -> ("error out"=w1053:errorcluster, "connection reference out"=w1048:T6)  [unwired: 5 in]
                  n828 = case shown="错误" w1053 {
                    selector: w1053 -> [w1055 w1076]
                    tunnel: w1050 -> [_ w1073]
                    tunnel: w1048 -> [w1056 w1065]
                    tunnel: w1052 -> [_ w1077]
                    tunnel: w1051 -> [_ w1069]
                    tunnel: [w1056 w1064] -> _
                    tunnel: [w1055 w1063] -> w1047
                    frame No Error {
                    }
                    frame Error {
                      n829 = Array Subset(array=w1073, index=3 ("长度"), length=2 ("长度")) -> (w1074:string[])
                      n830 = Unbundle(w1069) -> (w1058:i64, w1061:i64, "电机工位生产结果"=w1068:string, "result string"=w1067:string)  [unwired: 1 out]
                      n831 = Number To Decimal String(number=w1061) -> (decimal integer string=w1062:string)  [unwired: 1 in]
                      n832 = Number To Decimal String(number=w1058) -> (decimal integer string=w1057:string)  [unwired: 1 in]
                      n833 = Concatenate Strings("WHERE CODE_ID =" ("condition"), w1062, "AND DEVICE_ID = ", w1057) -> (w1070:string)
                      n834 = Bundle("电机工位生产结果"=w1068, "result string"=w1067) -> (w1066:T10)  [unwired: 1 in]
                      n835 = call <vilib>:"Clear Errors.vi"("error in (no error)"=w1076) -> ("error out"=w1075:errorcluster)  [unwired: 5 in, 1 out]
                      n836 = call <vilib>:"DB Tools Update Data.vi"("condition"=w1070, "data"=w1066, "error in (no error)"=w1075, "columns"=w1074, "table"=w1077, "connection reference"=w1065) -> ("error out"=w1063:errorcluster, "connection reference out"=w1064:T6)  [unwired: 4 in]
                    }
                  }
                }
                n837 = call <vilib>:"Simple Error Handler.vi"("error in (no error)"=w1044) -> ()  [unwired: 4 in, 5 out]
              }
              frame #1 {
                n838 = shared-variable "我的电脑\\Global.lvlib\\工位追溯码"() -> ()  [unwired: 1 in, 2 out]
                n839 = global read "Global1.vi" "电机码"() -> (w1078:string)
                n840 = global read "Global1.vi" "CODE_ID"() -> (w1079:string)
                n841 = Format Into String(format string="UPDATE\ndbo.[Code]\nSET dbo.[Code].CODE_MOTOR = '%s'\n\nWHERE\ndbo.[Code].CODE_ID = %s\n" ("格式字符串"), w1078, w1079) -> (resulting string=w1082:string)  [unwired: 2 in, 1 out]
                n842 = call "SQL_query.vi"("SQL query"=w1082, "联机模式"=enum16{"单机", "联网"}."联网") -> ()  [unwired: 1 in, 3 out]
              }
              frame #2 {
                n843 = local write "STEP3"("初始化" ("STEP")) -> ()
                n844 = call "浮动通知.vi"("通知内容"="电机工位数据录入成功！" ("Status")) -> ()  [unwired: 11 in]
                n845 = Wait (ms)(milliseconds to wait=u32 500 ("等待时间（毫秒）")) -> ()  [unwired: 1 out]
              }
            }
          }
          frame "不合格锁定" {
            n846 = call "临时授权.vi"() -> ("授权成功"=w1087:bool)  [unwired: 11 in]
            n847 = case shown="真" w1087 {
              frame False {
              }
              frame True {
                n848 = local write "STEP3"("报表" ("STEP")) -> ()
                n849 = shared-variable "我的电脑\\A17031611.lvlib\\设备状态1"(i16 3722 ("设备状态")) -> ()  [unwired: 1 in, 1 out]
              }
            }
            n850 = Wait (ms)(milliseconds to wait=u32 100 ("等待时间（毫秒）")) -> ()  [unwired: 1 out]
          }
          frame "报表" {
            n851 = call "浮动通知.vi"("通知内容"="报表生成中" ("Status")) -> ()  [unwired: 11 in]
            n852 = shared-variable "我的电脑\\Global.lvlib\\工位追溯码"() -> (w1099:string)  [unwired: 1 in, 1 out]
            n853 = Index Array(array="判定结果", index (col)=1 ("禁用的索引 (列)")) -> (element=w1094:bool[])  [unwired: 1 in]
            n854 = And Array Elements(Boolean array=w1094) -> (logical AND=w1091:bool)
            n855 = shared-variable "我的电脑\\Global.lvlib\\联机模式"() -> (w1096:i16)  [unwired: 1 in, 1 out]
            n856 = call "Report_A170316-11.vi"("文件重命名"=TRUE, "文件名称"=w1099, "布尔数组"="判定结果") -> ("error out"=w1097:errorcluster)  [unwired: 8 in]
            n857 = case shown="真" w1091 {
              frame False {
              }
              frame True {
                n858 = global read "Global.vi" "电机生产数量"() -> (w1108:refnum<vi>)
                n859 = property class="Num"(reference=w1108) -> (reference out=w1107:refnum<vi>, error out=w1106:errorcluster, "Value"=w1105:variant)  [unwired: 1 in]
                n860 = Variant To Data(type=u32 0, Variant=w1105) -> (data=w1104:u32)  [unwired: 1 in, 1 out]
                n861 = Increment(x=w1104) -> (x+1=w1103:u32)
                n862 = property class="Num"(reference=w1107, error in=w1106, "Value"=w1103) -> ()  [unwired: 2 out]
              }
            }
            n863 = case shown="0, 默认" w1096 {
              tunnel: w1097 -> [_ w1109]
              frame 0, Default {
              }
              frame 1 {
                n864 = call "上传数据库.vi"("错误输入"=w1109) -> ()  [unwired: 10 in, 1 out]
              }
            }
            n865 = shared-variable "我的电脑\\A17031611.lvlib\\设备状态1"() -> (w1090:i16)  [unwired: 1 in, 1 out]
            n866 = case shown="3721..3723" w1090 {
              frame Default {
                n867 = local write "STEP3"("初始化" ("STEP")) -> ()
              }
              frame 3721..3723 {
                n868 = local write "STEP3"("等待" ("STEP")) -> ()
              }
            }
          }
          frame "步骤" {
            n869 = case shown="\"安装弹簧\", 默认" "电机步骤" {
              selector: "电机步骤" -> [w1113 _]
              tunnel: [w1112 "等待"] -> w1110
              frame "安装弹簧", Default {
                n870 = global read "Global.vi" "电机安装"() -> (w1115:bool[])
                n871 = Index Array(array=w1115, index=w1113) -> (element=w1114:bool)
                n872 = case shown="真" w1114 {
                  tunnel: w1113 -> [_ w1121]
                  tunnel: ["步骤" w1120] -> w1112
                  frame False {
                    n873 = Wait (ms)(milliseconds to wait=u32 100 ("等待时间（毫秒）")) -> ()  [unwired: 1 out]
                    n874 = local read "电机步骤"() -> (w1119:T3)
                    n875 = Increment(x=w1119) -> (x+1=w1118:T3)
                    n876 = local write "电机步骤"(w1118) -> ()
                  }
                  frame True {
                    n877 = case shown="\"电机螺栓2\"" w1121 {
                      tunnel: ["等待" "等待" "等待" "等待" "等待" "等待" "等待" "等待" "等待"] -> w1120
                      frame "安装弹簧", Default {
                        n878 = shared-variable "我的电脑\\A17031611.lvlib\\设备状态3"(i16 16 ("设备状态")) -> ()  [unwired: 1 in, 1 out]
                      }
                      frame "安装O型圈" {
                        n879 = shared-variable "我的电脑\\A17031611.lvlib\\设备状态3"(i16 18 ("设备状态")) -> ()  [unwired: 1 in, 1 out]
                      }
                      frame "安装弹性垫圈" {
                        n880 = shared-variable "我的电脑\\A17031611.lvlib\\设备状态3"(i16 20 ("设备状态")) -> ()  [unwired: 1 in, 1 out]
                      }
                      frame "电机螺栓1" {
                        n881 = shared-variable "我的电脑\\A17031611.lvlib\\设备状态3"(i16 40 ("设备状态3")) -> ()  [unwired: 1 in, 1 out]
                      }
                      frame "电机螺栓2" {
                        n882 = shared-variable "我的电脑\\A17031611.lvlib\\设备状态3"(i16 42 ("设备状态控制字")) -> ()  [unwired: 1 in, 1 out]
                      }
                      frame "电机螺栓3" {
                        n883 = shared-variable "我的电脑\\A17031611.lvlib\\设备状态3"(i16 44 ("设备状态控制字")) -> ()  [unwired: 1 in, 1 out]
                      }
                      frame "电机拍照" {
                        n884 = shared-variable "我的电脑\\A17031611.lvlib\\设备状态3"(i16 70 ("设备状态控制字")) -> ()  [unwired: 1 in, 1 out]
                      }
                      frame "涂色标" {
                        n885 = shared-variable "我的电脑\\A17031611.lvlib\\设备状态3"(i16 90 ("设备状态控制字")) -> ()  [unwired: 1 in, 1 out]
                      }
                      frame "安装轧带取走工件" {
                        n886 = shared-variable "我的电脑\\A17031611.lvlib\\设备状态3"(i16 100 ("设备状态控制字")) -> ()  [unwired: 1 in, 1 out]
                      }
                    }
                  }
                }
              }
              frame "完成" {
                n887 = shared-variable "我的电脑\\A17031611.lvlib\\设备状态3"(i16 200 ("设备状态控制字")) -> ()  [unwired: 1 in, 1 out]
              }
            }
            n888 = local write "STEP3"(w1110) -> ()
          }
        }
        n889 = Wait (ms)(milliseconds to wait=u32 50 ("等待时间（毫秒）")) -> ()  [unwired: 1 out]
        n890 = global read "Global.vi" "程序关闭"() -> (w644:bool)
      }
      n891 = while {
        stop <- w1143 stop-if-true
        n892 = global read "Global.vi" "产品型号"() -> (w1144:string)
        n893 = call "Is Value Changed.vim"("value"=w1144) -> ("changed or first call?"=w1145:bool)
        n894 = event shown="[2] \"更换产品\": 值改变" {
          selector: _ -> [_ _ _ _]
          dyn-events: _ -> [_ _ _ _]
          timeout: 5 -> [_ _ _ _]
          tunnel: w1144 -> [_ w1164 w1449 _]
          event Timeout {
            n895 = event-data() -> ()  [unwired: 1 in, 3 out]
            n896 = shared-variable "我的电脑\\A17031611.lvlib\\错误代码"() -> (w1148:u16)  [unwired: 1 in, 1 out]
            n897 = feedback #1() -> (w1158:u16)  [unwired: 1 in]
            n898 = feedback-in #1(w1148) -> ()
            n899 = Greater Or Equal?(x=w1148, y=i16 5000) -> (x >= y?=w1156:bool)
            n900 = Less?(x=w1148, y=i16 5200) -> (x < y?=w1157:bool)
            n901 = Equal?(x=w1148, y=w1158) -> (x = y?=w1155:bool)
            n902 = global read "Global.vi" "报警图标"() -> (w1150:refnum<vi>)
            n903 = And(x=w1156, y=w1157) -> (x .and. y?=w1149:bool)
            n904 = property class="Bool"(reference=w1150, "Value"=w1149) -> ()  [unwired: 1 in, 2 out]
            n905 = Bundle By Name(cluster=errorcluster {"status"=FALSE, "code"=0, "source"=""} ("错误常量"), "status"=w1149, "code"=w1148) -> (w1154:errorcluster)
            n906 = case shown="真" w1155 {
              tunnel: w1154 -> [w1163 _]
              frame False {
                n907 = call "报警处理.vi"("错误常量"=w1163) -> ()  [unwired: 9 in, 2 out]
              }
              frame True {
              }
            }
            n908 = case shown="0" w1148 {
              frame 0 {
                n909 = global read "Global.vi" "报警图标"() -> (w1159:refnum<vi>)
                n910 = property class="Bool"(reference=w1159, "Visible"=FALSE ("可见")) -> ()  [unwired: 1 in, 2 out]
              }
              frame 1, Default {
                n911 = global read "Global.vi" "报警图标"() -> (w1162:refnum<vi>)
                n912 = property class="Bool"(reference=w1162, "Visible"=TRUE ("可见")) -> ()  [unwired: 1 in, 2 out]
              }
            }
          }
          event "前序OK？": Value Change {
            n913 = event-data() -> ()  [unwired: 1 in, 6 out]
            n914 = stacked-sequence {
              tunnel: w1164 -> [_ w1218]
              frame #0 {
                n915 = disable-structure shown="禁用" {
                  frame Disabled {
                    n916 = control-ref of="安装扎带并取走工件"() -> (w1171:refnum<vi>)
                    n917 = control-ref of="安装扎带和线卡并取走工件"() -> (w1170:refnum<vi>)
                    n918 = control-ref of="控制器安装螺栓1拧紧确认"() -> (w1191:refnum<vi>)
                    n919 = control-ref of="控制器安装螺栓2拧紧确认"() -> (w1188:refnum<vi>)
                    n920 = control-ref of="安装支架涂色标"() -> (w1190:refnum<vi>)
                    n921 = control-ref of="安装支架扎带安装"() -> (w1174:refnum<vi>)
                    n922 = control-ref of="安装支架线卡扎带安装"() -> (w1173:refnum<vi>)
                    n923 = control-ref of="控制器安装螺栓3拧紧确认"() -> (w1169:refnum<vi>)
                    n924 = control-ref of="安装支架螺栓1拧紧确认"() -> (w1193:refnum<vi>)
                    n925 = control-ref of="安装支架螺栓4拧紧确认"() -> (w1165:refnum<vi>)
                    n926 = control-ref of="安装弹性垫圈弹簧并按启动拍照"() -> (w1180:refnum<vi>)
                    n927 = control-ref of="安装扎带并取走工件"() -> (w1175:refnum<vi>)
                    n928 = control-ref of="电机安装螺栓2扭矩确认"() -> (w1178:refnum<vi>)
                    n929 = control-ref of="安装支架螺栓3拧紧确认"() -> (w1168:refnum<vi>)
                    n930 = control-ref of="安装支架螺栓2拧紧确认"() -> (w1192:refnum<vi>)
                    n931 = control-ref of="电机安装螺栓3扭矩确认"() -> (w1166:refnum<vi>)
                    n932 = control-ref of="按启动按钮拍照确认"() -> (w1177:refnum<vi>)
                    n933 = control-ref of="电机安装螺栓1扭矩确认"() -> (w1179:refnum<vi>)
                    n934 = control-ref of="控制器支架涂色标"() -> (w1182:refnum<vi>)
                    n935 = control-ref of="涂色标"() -> (w1176:refnum<vi>)
                    n936 = Build Array(w1193, w1192, w1191, w1188, w1190, w1174, w1173, w1169, w1168, w1165) -> (w1189:refnum<vi>[])
                    n937 = control-ref of="控制器支架螺栓1拧紧确认"() -> (w1186:refnum<vi>)
                    n938 = control-ref of="控制器支架螺栓3拧紧确认"() -> (w1184:refnum<vi>)
                    n939 = for {
                      tunnel: w1189 -> [w1217] mode=indexing
                      i -> [w1216]
                      n940 = Multiply(x=60, y=w1216) -> (x*y=w1211:i32)
                      n941 = Add(x=340 ("y"), y=w1211) -> (x+y=w1213:i32)
                      n942 = Bundle("y"=-500, w1213) -> (w1212:cluster{"y":i32, i32})  [unwired: 1 in]
                      n943 = property class="Bool (严格)"(reference=w1217, "Position"=w1212) -> ()  [unwired: 1 in, 2 out]
                    }
                    n944 = control-ref of="控制器支架安装线卡扎带"() -> (w1172:refnum<vi>)
                    n945 = control-ref of="控制器支架螺栓4拧紧确认"() -> (w1183:refnum<vi>)
                    n946 = Build Array(w1180, w1179, w1178, w1177, w1176, w1175, w1171, w1170, w1166) -> (w1181:refnum<vi>[])
                    n947 = control-ref of="控制器支架螺栓2拧紧确认"() -> (w1185:refnum<vi>)
                    n948 = control-ref of="控制器支架螺栓5拧紧确认"() -> (w1167:refnum<vi>)
                    n949 = for {
                      tunnel: w1181 -> [w1201] mode=indexing
                      i -> [w1200]
                      n950 = Multiply(x=60, y=w1200) -> (x*y=w1198:i32)
                      n951 = Add(x=w1198, y=340) -> (x+y=w1195:i32)
                      n952 = Bundle("y"=-1500, w1195) -> (w1194:cluster{"y":i32, i32})  [unwired: 1 in]
                      n953 = property class="Bool (严格)"(reference=w1201, "Position"=w1194) -> ()  [unwired: 1 in, 2 out]
                    }
                    n954 = Build Array(w1186, w1185, w1184, w1183, w1182, w1172, w1167) -> (w1187:refnum<vi>[])
                    n955 = for {
                      tunnel: w1187 -> [w1209] mode=indexing
                      i -> [w1208]
                      n956 = Multiply(x=60, y=w1208) -> (x*y=w1206:i32)
                      n957 = Add(x=w1206, y=345) -> (x+y=w1203:i32)
                      n958 = Bundle("y"=-1000, w1203) -> (w1202:cluster{"y":i32, i32})  [unwired: 1 in]
                      n959 = property class="Bool (严格)"(reference=w1209, "Position"=w1202) -> ()  [unwired: 1 in, 2 out]
                    }
                  }
                  frame Enabled {
                  }
                }
              }
              frame #1 {
                n960 = disable-structure shown="禁用" {
                  disable-tunnel: w1218 -> [w1219 _]
                  frame Disabled {
                    n961 = case shown="\"R092B\"" w1219 {
                      frame Default {
                      }
                      frame "R92A" {
                        n962 = control-ref of="控制器安装螺栓2拧紧确认"() -> (w1224:refnum<vi>)
                        n963 = control-ref of="安装支架螺栓4拧紧确认"() -> (w1226:refnum<vi>)
                        n964 = control-ref of="控制器安装螺栓1拧紧确认"() -> (w1225:refnum<vi>)
                        n965 = control-ref of="安装支架螺栓1拧紧确认"() -> (w1229:refnum<vi>)
                        n966 = control-ref of="安装支架螺栓3拧紧确认"() -> (w1227:refnum<vi>)
                        n967 = control-ref of="控制器安装螺栓3拧紧确认"() -> (w1223:refnum<vi>)
                        n968 = control-ref of="安装支架涂色标"() -> (w1222:refnum<vi>)
                        n969 = control-ref of="安装支架螺栓2拧紧确认"() -> (w1228:refnum<vi>)
                        n970 = control-ref of="安装弹性垫圈弹簧并按启动拍照"() -> (w1236:refnum<vi>)
                        n971 = control-ref of="电机安装螺栓3扭矩确认"() -> (w1230:refnum<vi>)
                        n972 = control-ref of="电机安装螺栓1扭矩确认"() -> (w1235:refnum<vi>)
                        n973 = control-ref of="电机安装螺栓2扭矩确认"() -> (w1234:refnum<vi>)
                        n974 = control-ref of="按启动按钮拍照确认"() -> (w1233:refnum<vi>)
                        n975 = control-ref of="安装扎带并取走工件"() -> (w1231:refnum<vi>)
                        n976 = Build Array(w1229, w1228, w1227, w1226, w1225, w1224, w1223, w1222) -> (w1221:refnum<vi>[])
                        n977 = control-ref of="涂色标"() -> (w1232:refnum<vi>)
                        n978 = for {
                          tunnel: w1221 -> [w1266] mode=indexing
                          i -> [w1265]
                          n979 = Multiply(x=60, y=w1265) -> (x*y=w1260:i32)
                          n980 = Add(x=340 ("y"), y=w1260) -> (x+y=w1262:i32)
                          n981 = Bundle("y"=1775, w1262) -> (w1261:cluster{"y":i32, i32})  [unwired: 1 in]
                          n982 = property class="Bool (严格)"(reference=w1266, "Position"=w1261) -> ()  [unwired: 1 in, 2 out]
                        }
                        n983 = Build Array(w1236, w1235, w1234, w1230, w1233, w1232, w1231) -> (w1237:refnum<vi>[])
                        n984 = control-ref of="控制器支架螺栓2拧紧确认"() -> (w1240:refnum<vi>)
                        n985 = control-ref of="控制器支架螺栓1拧紧确认"() -> (w1241:refnum<vi>)
                        n986 = control-ref of="控制器支架螺栓3拧紧确认"() -> (w1239:refnum<vi>)
                        n987 = control-ref of="控制器支架螺栓4拧紧确认"() -> (w1238:refnum<vi>)
                        n988 = control-ref of="控制器支架涂色标"() -> (w1220:refnum<vi>)
                        n989 = for {
                          tunnel: w1237 -> [w1250] mode=indexing
                          i -> [w1249]
                          n990 = Multiply(x=60, y=w1249) -> (x*y=w1247:i32)
                          n991 = Add(x=w1247, y=340) -> (x+y=w1244:i32)
                          n992 = Bundle("y"=2115, w1244) -> (w1243:cluster{"y":i32, i32})  [unwired: 1 in]
                          n993 = property class="Bool (严格)"(reference=w1250, "Position"=w1243) -> ()  [unwired: 1 in, 2 out]
                        }
                        n994 = Build Array(w1241, w1240, w1239, w1238, w1220) -> (w1242:refnum<vi>[])
                        n995 = for {
                          tunnel: w1242 -> [w1258] mode=indexing
                          i -> [w1257]
                          n996 = Multiply(x=60, y=w1257) -> (x*y=w1255:i32)
                          n997 = Add(x=w1255, y=345) -> (x+y=w1252:i32)
                          n998 = Bundle("y"=1445, w1252) -> (w1251:cluster{"y":i32, i32})  [unwired: 1 in]
                          n999 = property class="Bool (严格)"(reference=w1258, "Position"=w1251) -> ()  [unwired: 1 in, 2 out]
                        }
                      }
                      frame "R128" {
                        # "1345"
                        n1000 = control-ref of="安装支架螺栓2拧紧确认"() -> (w1282:refnum<vi>)
                        n1001 = control-ref of="安装支架涂色标"() -> (w1281:refnum<vi>)
                        n1002 = control-ref of="安装支架螺栓1拧紧确认"() -> (w1283:refnum<vi>)
                        n1003 = control-ref of="控制器安装螺栓1拧紧确认"() -> (w1285:refnum<vi>)
                        n1004 = control-ref of="控制器安装螺栓2拧紧确认"() -> (w1284:refnum<vi>)
                        n1005 = control-ref of="安装弹性垫圈弹簧并按启动拍照"() -> (w1276:refnum<vi>)
                        n1006 = control-ref of="电机安装螺栓1扭矩确认"() -> (w1275:refnum<vi>)
                        n1007 = control-ref of="电机安装螺栓2扭矩确认"() -> (w1274:refnum<vi>)
                        n1008 = control-ref of="涂色标"() -> (w1272:refnum<vi>)
                        n1009 = control-ref of="安装扎带并取走工件"() -> (w1271:refnum<vi>)
                        n1010 = control-ref of="按启动按钮拍照确认"() -> (w1273:refnum<vi>)
                        n1011 = Build Array(w1285, w1284, w1283, w1282, w1281) -> (w1288:refnum<vi>[])
                        n1012 = control-ref of="控制器支架螺栓2拧紧确认"() -> (w1279:refnum<vi>)
                        n1013 = control-ref of="控制器支架螺栓1拧紧确认"() -> (w1280:refnum<vi>)
                        n1014 = control-ref of="控制器支架螺栓3拧紧确认"() -> (w1278:refnum<vi>)
                        n1015 = control-ref of="控制器支架螺栓5拧紧确认"() -> ()  [unwired: 1 out]
                        n1016 = control-ref of="控制器支架涂色标"() -> (w1270:refnum<vi>)
                        n1017 = control-ref of="控制器支架螺栓4拧紧确认"() -> (w1277:refnum<vi>)
                        n1018 = for {
                          tunnel: w1288 -> [w1320] mode=indexing
                          i -> [w1319]
                          n1019 = Multiply(x=60, y=w1319) -> (x*y=w1314:i32)
                          n1020 = Add(x=438 ("y"), y=w1314) -> (x+y=w1316:i32)
                          n1021 = Bundle("y"=-1495, w1316) -> (w1315:cluster{"y":i32, i32})  [unwired: 1 in]
                          n1022 = property class="Bool (严格)"(reference=w1320, "Position"=w1315) -> ()  [unwired: 1 in, 2 out]
                        }
                        n1023 = Build Array(w1276, w1275, w1274, w1273, w1272, w1271) -> (w1286:refnum<vi>[])
                        n1024 = for {
                          tunnel: w1286 -> [w1304] mode=indexing
                          i -> [w1303]
                          n1025 = Multiply(x=60, y=w1303) -> (x*y=w1301:i32)
                          n1026 = Add(x=w1301, y=438) -> (x+y=w1298:i32)
                          n1027 = Bundle("y"=-1145, w1298) -> (w1297:cluster{"y":i32, i32})  [unwired: 1 in]
                          n1028 = property class="Bool (严格)"(reference=w1304, "Position"=w1297) -> ()  [unwired: 1 in, 2 out]
                        }
                        n1029 = control-ref of="安装支架螺栓3拧紧确认"() -> (w1269:refnum<vi>)
                        n1030 = Build Array(w1280, w1279, w1278, w1277, w1270) -> (w1287:refnum<vi>[])
                        n1031 = control-ref of="安装支架螺栓4拧紧确认"() -> (w1267:refnum<vi>)
                        n1032 = for {
                          tunnel: w1287 -> [w1312] mode=indexing
                          i -> [w1311]
                          n1033 = Multiply(x=60, y=w1311) -> (x*y=w1309:i32)
                          n1034 = Add(x=w1309, y=438) -> (x+y=w1306:i32)
                          n1035 = Bundle("y"=-1820, w1306) -> (w1305:cluster{"y":i32, i32})  [unwired: 1 in]
                          n1036 = property class="Bool (严格)"(reference=w1312, "Position"=w1305) -> ()  [unwired: 1 in, 2 out]
                        }
                        n1037 = Build Array(w1269, w1267) -> (w1268:refnum<vi>[])
                        n1038 = for {
                          tunnel: w1268 -> [w1296] mode=indexing
                          i -> [w1295]
                          n1039 = Multiply(x=60, y=w1295) -> (x*y=w1293:i32)
                          n1040 = Add(x=w1293, y=438) -> (x+y=w1290:i32)
                          n1041 = Bundle("y"=-100, w1290) -> (w1289:cluster{"y":i32, i32})  [unwired: 1 in]
                          n1042 = property class="Bool (严格)"(reference=w1296, "Position"=w1289) -> ()  [unwired: 1 in, 2 out]
                        }
                      }
                      frame "R092B" {
                        # "1345"
                        n1043 = control-ref of="安装支架螺栓3拧紧确认"() -> (w1321:refnum<vi>)
                        n1044 = control-ref of="安装支架涂色标"() -> (w1333:refnum<vi>)
                        n1045 = control-ref of="安装支架螺栓2拧紧确认"() -> (w1334:refnum<vi>)
                        n1046 = control-ref of="安装支架螺栓1拧紧确认"() -> (w1335:refnum<vi>)
                        n1047 = control-ref of="控制器安装螺栓1拧紧确认"() -> (w1337:refnum<vi>)
                        n1048 = control-ref of="控制器安装螺栓2拧紧确认"() -> (w1336:refnum<vi>)
                        n1049 = control-ref of="安装弹性垫圈弹簧并按启动拍照"() -> (w1328:refnum<vi>)
                        n1050 = control-ref of="电机安装螺栓1扭矩确认"() -> (w1327:refnum<vi>)
                        n1051 = control-ref of="电机安装螺栓2扭矩确认"() -> (w1326:refnum<vi>)
                        n1052 = control-ref of="涂色标"() -> (w1324:refnum<vi>)
                        n1053 = control-ref of="安装扎带并取走工件"() -> (w1323:refnum<vi>)
                        n1054 = control-ref of="按启动按钮拍照确认"() -> (w1325:refnum<vi>)
                        n1055 = Build Array(w1337, w1336, w1335, w1334, w1321, w1333) -> (w1340:refnum<vi>[])
                        n1056 = control-ref of="控制器支架螺栓2拧紧确认"() -> (w1331:refnum<vi>)
                        n1057 = control-ref of="控制器支架螺栓1拧紧确认"() -> (w1332:refnum<vi>)
                        n1058 = control-ref of="控制器支架螺栓3拧紧确认"() -> (w1330:refnum<vi>)
                        n1059 = control-ref of="控制器支架涂色标"() -> (w1322:refnum<vi>)
                        n1060 = control-ref of="控制器支架螺栓4拧紧确认"() -> (w1329:refnum<vi>)
                        n1061 = for {
                          tunnel: w1340 -> [w1364] mode=indexing
                          i -> [w1363]
                          n1062 = Multiply(x=60, y=w1363) -> (x*y=w1358:i32)
                          n1063 = Add(x=438 ("y"), y=w1358) -> (x+y=w1360:i32)
                          n1064 = Bundle("y"=-1495, w1360) -> (w1359:cluster{"y":i32, i32})  [unwired: 1 in]
                          n1065 = property class="Bool (严格)"(reference=w1364, "Position"=w1359) -> ()  [unwired: 1 in, 2 out]
                        }
                        n1066 = Build Array(w1328, w1327, w1326, w1325, w1324, w1323) -> (w1338:refnum<vi>[])
                        n1067 = for {
                          tunnel: w1338 -> [w1348] mode=indexing
                          i -> [w1347]
                          n1068 = Multiply(x=60, y=w1347) -> (x*y=w1345:i32)
                          n1069 = Add(x=w1345, y=438) -> (x+y=w1342:i32)
                          n1070 = Bundle("y"=-1145, w1342) -> (w1341:cluster{"y":i32, i32})  [unwired: 1 in]
                          n1071 = property class="Bool (严格)"(reference=w1348, "Position"=w1341) -> ()  [unwired: 1 in, 2 out]
                        }
                        n1072 = Build Array(w1332, w1331, w1330, w1329, w1322) -> (w1339:refnum<vi>[])
                        n1073 = control-ref of="控制器支架螺栓5拧紧确认"() -> ()  [unwired: 1 out]
                        n1074 = for {
                          tunnel: w1339 -> [w1356] mode=indexing
                          i -> [w1355]
                          n1075 = Multiply(x=60, y=w1355) -> (x*y=w1353:i32)
                          n1076 = Add(x=w1353, y=438) -> (x+y=w1350:i32)
                          n1077 = Bundle("y"=-1820, w1350) -> (w1349:cluster{"y":i32, i32})  [unwired: 1 in]
                          n1078 = property class="Bool (严格)"(reference=w1356, "Position"=w1349) -> ()  [unwired: 1 in, 2 out]
                        }
                      }
                      frame "R563X" {
                        # "1345"
                        n1079 = control-ref of="安装支架螺栓2拧紧确认"() -> (w1384:refnum<vi>)
                        n1080 = control-ref of="安装支架涂色标"() -> (w1383:refnum<vi>)
                        n1081 = control-ref of="安装支架螺栓1拧紧确认"() -> (w1385:refnum<vi>)
                        n1082 = control-ref of="控制器安装螺栓1拧紧确认"() -> (w1387:refnum<vi>)
                        n1083 = control-ref of="控制器安装螺栓2拧紧确认"() -> (w1386:refnum<vi>)
                        n1084 = control-ref of="安装弹性垫圈弹簧并按启动拍照"() -> (w1379:refnum<vi>)
                        n1085 = control-ref of="电机安装螺栓1扭矩确认"() -> (w1378:refnum<vi>)
                        n1086 = control-ref of="电机安装螺栓2扭矩确认"() -> (w1377:refnum<vi>)
                        n1087 = control-ref of="涂色标"() -> (w1375:refnum<vi>)
                        n1088 = control-ref of="安装扎带并取走工件"() -> (w1374:refnum<vi>)
                        n1089 = control-ref of="按启动按钮拍照确认"() -> (w1376:refnum<vi>)
                        n1090 = control-ref of="控制器支架螺栓2拧紧确认"() -> (w1381:refnum<vi>)
                        n1091 = control-ref of="控制器支架螺栓1拧紧确认"() -> (w1382:refnum<vi>)
                        n1092 = control-ref of="控制器支架螺栓3拧紧确认"() -> (w1380:refnum<vi>)
                        n1093 = control-ref of="控制器支架涂色标"() -> (w1373:refnum<vi>)
                        n1094 = Build Array(w1387, w1386, w1385, w1384, w1383) -> (w1390:refnum<vi>[])
                        n1095 = control-ref of="控制器支架螺栓5拧紧确认"() -> (w1368:refnum<vi>)
                        n1096 = control-ref of="控制器支架螺栓4拧紧确认"() -> (w1367:refnum<vi>)
                        n1097 = control-ref of="安装支架线卡扎带安装"() -> (w1366:refnum<vi>)
                        n1098 = for {
                          tunnel: w1390 -> [w1422] mode=indexing
                          i -> [w1421]
                          n1099 = Multiply(x=60, y=w1421) -> (x*y=w1416:i32)
                          n1100 = Add(x=438 ("y"), y=w1416) -> (x+y=w1418:i32)
                          n1101 = Bundle("y"=-1495, w1418) -> (w1417:cluster{"y":i32, i32})  [unwired: 1 in]
                          n1102 = property class="Bool (严格)"(reference=w1422, "Position"=w1417) -> ()  [unwired: 1 in, 2 out]
                        }
                        n1103 = Build Array(w1379, w1378, w1377, w1376, w1375, w1374) -> (w1388:refnum<vi>[])
                        n1104 = control-ref of="安装支架扎带安装"() -> (w1369:refnum<vi>)
                        n1105 = control-ref of="安装扎带和线卡并取走工件"() -> (w1370:refnum<vi>)
                        n1106 = control-ref of="控制器支架安装线卡扎带"() -> ()  [unwired: 1 out]
                        n1107 = control-ref of="控制器支架螺栓5拧紧确认"() -> (w1371:refnum<vi>)
                        n1108 = control-ref of="控制器支架螺栓4拧紧确认"() -> (w1372:refnum<vi>)
                        n1109 = for {
                          tunnel: w1388 -> [w1406] mode=indexing
                          i -> [w1405]
                          n1110 = Multiply(x=60, y=w1405) -> (x*y=w1403:i32)
                          n1111 = Add(x=w1403, y=438) -> (x+y=w1400:i32)
                          n1112 = Bundle("y"=-1145, w1400) -> (w1399:cluster{"y":i32, i32})  [unwired: 1 in]
                          n1113 = property class="Bool (严格)"(reference=w1406, "Position"=w1399) -> ()  [unwired: 1 in, 2 out]
                        }
                        n1114 = Build Array(w1382, w1381, w1380, w1373) -> (w1389:refnum<vi>[])
                        n1115 = Build Array(w1372, w1371, w1370, w1369, w1368, w1367, w1366) -> (w1365:refnum<vi>[])
                        n1116 = for {
                          tunnel: w1389 -> [w1414] mode=indexing
                          i -> [w1413]
                          n1117 = Multiply(x=60, y=w1413) -> (x*y=w1411:i32)
                          n1118 = Add(x=w1411, y=438) -> (x+y=w1408:i32)
                          n1119 = Bundle("y"=-1820, w1408) -> (w1407:cluster{"y":i32, i32})  [unwired: 1 in]
                          n1120 = property class="Bool (严格)"(reference=w1414, "Position"=w1407) -> ()  [unwired: 1 in, 2 out]
                        }
                        n1121 = for {
                          tunnel: w1365 -> [w1398] mode=indexing
                          i -> [w1397]
                          n1122 = Multiply(x=60, y=w1397) -> (x*y=w1395:i32)
                          n1123 = Add(x=w1395, y=438) -> (x+y=w1392:i32)
                          n1124 = Bundle("y"=-100, w1392) -> (w1391:cluster{"y":i32, i32})  [unwired: 1 in]
                          n1125 = property class="Bool (严格)"(reference=w1398, "Position"=w1391) -> ()  [unwired: 1 in, 2 out]
                        }
                      }
                    }
                  }
                  frame Enabled {
                  }
                }
              }
            }
          }
          event "更换产品": Value Change {
            n1126 = event-data() -> ()  [unwired: 1 in, 6 out]
            n1127 = control-ref of="控制器支架安装线卡扎带"() -> (w1451:refnum<vi>)
            n1128 = control-ref of="控制器支架螺栓5拧紧确认"() -> (w1453:refnum<vi>)
            n1129 = control-ref of="控制器支架涂色标"() -> (w1452:refnum<vi>)
            n1130 = control-ref of="控制器支架螺栓3拧紧确认"() -> (w1455:refnum<vi>)
            n1131 = control-ref of="控制器支架螺栓4拧紧确认"() -> (w1454:refnum<vi>)
            n1132 = control-ref of="控制器支架螺栓2拧紧确认"() -> (w1456:refnum<vi>)
            n1133 = control-ref of="控制器支架螺栓1拧紧确认"() -> (w1457:refnum<vi>)
            n1134 = control-ref of="安装支架螺栓4拧紧确认"() -> (w1441:refnum<vi>)
            n1135 = global read "Global.vi" "控制器支架"() -> (w1448:bool[])
            n1136 = control-ref of="安装支架线卡扎带安装"() -> ()  [unwired: 1 out]
            n1137 = control-ref of="安装支架螺栓2拧紧确认"() -> (w1443:refnum<vi>)
            n1138 = control-ref of="安装支架螺栓3拧紧确认"() -> (w1442:refnum<vi>)
            n1139 = control-ref of="安装支架涂色标"() -> (w1440:refnum<vi>)
            n1140 = control-ref of="安装扎带和线卡并取走工件"() -> (w1439:refnum<vi>)
            n1141 = control-ref of="控制器安装螺栓2拧紧确认"() -> (w1446:refnum<vi>)
            n1142 = control-ref of="安装支架螺栓1拧紧确认"() -> (w1444:refnum<vi>)
            n1143 = control-ref of="控制器安装螺栓3拧紧确认"() -> (w1445:refnum<vi>)
            n1144 = control-ref of="控制器安装螺栓1拧紧确认"() -> (w1447:refnum<vi>)
            n1145 = Build Array(w1457, w1456, w1455, w1454, w1453, w1452, w1451) -> (w1425:refnum<vi>[])
            n1146 = for "For循环" {
              tunnel: w1448 -> [w1491] mode=indexing
              tunnel: w1425 -> [w1490] mode=indexing
              shift-right: [w1488] -> _
              shift-left: 360 -> [w1489]
              tunnel: w1425 -> [w1487]
              i -> [w1486]
              n1147 = case shown="假" w1491 {
                tunnel: w1490 -> [w1493 w1495]
                tunnel: w1489 -> [w1494 w1500]
                tunnel: [w1494 w1497] -> w1488
                tunnel: w1487 -> [_ _]
                tunnel: w1486 -> [_ _]
                frame False {
                  n1148 = property class="Bool (严格)"(reference=w1493, "Top"=-100 ("位置:置顶")) -> ()  [unwired: 1 in, 2 out]
                }
                frame True {
                  n1149 = Add(x=w1500, y=50) -> (x+y=w1497:i32)
                  n1150 = Bundle(-1850, w1497) -> (w1498:cluster{i32, i32})  [unwired: 1 in]
                  n1151 = property class="Bool (严格)"(reference=w1495, "Position"=w1498) -> ()  [unwired: 1 in, 2 out]
                }
              }
            }
            n1152 = global read "Global.vi" "控制器安装支架"() -> (w1438:bool[])
            n1153 = Build Array(w1447, w1446, w1445, w1444, w1443, w1442, w1441, w1440, w1439) -> (w1437:refnum<vi>[])
            n1154 = for "For循环" {
              tunnel: w1438 -> [w1476] mode=indexing
              tunnel: w1437 -> [w1475] mode=indexing
              shift-right: [w1473] -> _
              shift-left: 360 -> [w1474]
              tunnel: w1437 -> [w1472]
              n1155 = case shown="真" w1476 {
                tunnel: w1475 -> [w1478 w1480]
                tunnel: w1474 -> [w1479 w1485]
                tunnel: [w1479 w1482] -> w1473
                tunnel: w1472 -> [_ _]
                frame False {
                  n1156 = property class="Bool (严格)"(reference=w1478, "Top"=-100 ("位置:置顶")) -> ()  [unwired: 1 in, 2 out]
                }
                frame True {
                  n1157 = Add(x=w1485, y=50) -> (x+y=w1482:i32)
                  n1158 = Bundle(-1510, w1482) -> (w1483:cluster{i32, i32})  [unwired: 1 in]
                  n1159 = property class="Bool (严格)"(reference=w1480, "Position"=w1483) -> ()  [unwired: 1 in, 2 out]
                }
              }
            }
            n1160 = control-ref of="电机安装螺栓1扭矩确认"() -> (w1434:refnum<vi>)
            n1161 = control-ref of="安装弹性垫圈弹簧并按启动拍照"() -> (w1435:refnum<vi>)
            n1162 = control-ref of="请拾取O型圈"() -> (w1424:refnum<vi>)
            n1163 = control-ref of="请拾取弹簧"() -> (w1423:refnum<vi>)
            n1164 = control-ref of="安装扎带并取走工件"() -> (w1429:refnum<vi>)
            n1165 = control-ref of="电机安装螺栓3扭矩确认"() -> (w1432:refnum<vi>)
            n1166 = control-ref of="电机安装螺栓2扭矩确认"() -> (w1433:refnum<vi>)
            n1167 = control-ref of="按启动按钮拍照确认"() -> (w1431:refnum<vi>)
            n1168 = control-ref of="安装支架扎带安装"() -> ()  [unwired: 1 out]
            n1169 = control-ref of="涂色标"() -> (w1430:refnum<vi>)
            n1170 = global read "Global.vi" "电机安装"() -> (w1427:bool[])
            n1171 = Build Array(w1423, w1424, w1435, w1434, w1433, w1432, w1431, w1430, w1429) -> (w1428:refnum<vi>[])
            n1172 = for "For循环" {
              tunnel: w1427 -> [w1462] mode=indexing
              tunnel: w1428 -> [w1461] mode=indexing
              shift-right: [w1459] -> _
              shift-left: 360 -> [w1460]
              tunnel: w1428 -> [w1458]
              n1173 = case shown="真" w1462 {
                tunnel: w1461 -> [w1464 w1466]
                tunnel: w1460 -> [w1465 w1471]
                tunnel: [w1465 w1468] -> w1459
                tunnel: w1458 -> [_ _]
                frame False {
                  n1174 = property class="Bool (严格)"(reference=w1464, "Top"=-100 ("位置:置顶")) -> ()  [unwired: 1 in, 2 out]
                }
                frame True {
                  n1175 = Add(x=w1471, y=50) -> (x+y=w1468:i32)
                  n1176 = Bundle(-1193, w1468) -> (w1469:cluster{i32, i32})  [unwired: 1 in]
                  n1177 = property class="Bool (严格)"(reference=w1466, "Position"=w1469) -> ()  [unwired: 1 in, 2 out]
                }
              }
            }
            "产品型号" <- w1449
          }
          event Panel Close {
            n1178 = event-data() -> ()  [unwired: 1 in, 4 out]
            n1179 = global write "Global.vi" "程序关闭"(TRUE ("程序关闭")) -> ()
          }
        }
        n1180 = case shown="真" w1145 {
          tunnel: w1144 -> [_ w1147]
          frame False {
          }
          frame True {
            n1181 = property on="更换布局" class="Str"("Val(Sgnl)"=w1147) -> ()  [unwired: 2 in, 2 out]
          }
        }
        n1182 = control-ref of="更换产品"() -> (w1142:refnum<vi>)
        n1183 = global write "Global.vi" "更换产品"(w1142) -> ()
        n1184 = global read "Global.vi" "程序关闭"() -> (w1143:bool)
      }
    }
  }
